vi "IE Default UI.vi"(10 "Color icon in":T4={"image type"=0, "image depth"=8, "image"=[255, 255, 255, 255, 255, 255, 255, 255, 255, 255, 255, 255, 255, 255, 255, 255, 255, 255, 255, 255, 255, 255, 255, 255, 255, 255, 255, 255, 255, 255, 255, 255, 255, 0, 0, 0, 0, 0, 0, 0, 0, 0, 0, 0, 0, 0, 0, 0, 0, 0, 0, 0, 0, 0, 0, 0, 0, 0, 0, 0, 0, 0, 0, 255, 255, 0, 0, 0, 0, 0, 0, 0, 0, 0, 0, 0, 0, 0, 0, 0, 0, 0, 0, 0, 0, 0, 0, 0, 0, 0, 0, 0, 0, 0, 0, 255, 255, 0, 0, 255, 255, 255, 255, 255, 255, 255, 255, 255, 255, 255, 255, 255, 255, 255, 255, 255, 255, 255, 0, 0, 0, 0, 0, 0, 0, 0, 0, 255, 255, 0, 0, 255, 250, 250, 250, 250, 250, 250, 250, 250, 250, 250, 250, 250, 248, 250, 44, 250, 44, 255, 0, 0, 0, 0, 0, 0, 0, 0, 0, 255, 255, 0, 0, 255, 250, 255, 255, 255, 255, 255, 255, 255, 255, 255, 255, 255, 248, 250, 44, 250, 44, 255, 0, 0, 0, 0, 0, 0, 0, 0, 0, 255, 255, 0, 0, 255, 250, 255, 209, 197, 209, 255, 255, 255, 209, 197, 209, 255, 248, 252, 43, 252, 44, 255, 0, 0, 0, 0, 0, 0, 0, 0, 0, 255, 255, 0, 0, 255, 250, 255, 197, 255, 197, 255, 255, 255, 197, 255, 197, 255, 248, 44, 44, 44, 44, 255, 0, 0, 0, 0, 0, 0, 0, 0, 0, 255, 255, 0, 0, 255, 250, 209, 197, 255, 197, 209, 255, 209, 197, 255, 197, 209, 248, 43, 252, 43, 44, 255, 0, 0, 0, 0, 0, 0, 0, 0, 0, 255, 255, 0, 0, 255, 250, 197, 209, 255, 209, 197, 255, 197, 209, 255, 209, 197, 248, 252, 8, 252, 44, 255, 0, 0, 0, 0, 0, 0, 0, 0, 0, 255, 255, 0, 0, 255, 250, 197, 255, 255, 255, 197, 255, 197, 255, 255, 255, 197, 248, 252, 8, 252, 44, 255, 0, 0, 0, 0, 0, 0, 0, 0, 0, 255, 255, 0, 0, 255, 250, 255, 255, 255, 255, 209, 197, 209, 255, 255, 255, 255, 248, 43, 252, 43, 44, 255, 0, 0, 0, 0, 0, 0, 0, 0, 0, 255, 255, 0, 0, 255, 250, 255, 255, 255, 255, 255, 255, 255, 255, 255, 255, 255, 248, 44, 44, 44, 44, 255, 0, 0, 0, 0, 0, 0, 0, 0, 0, 255, 255, 0, 0, 255, 248, 248, 248, 248, 248, 248, 248, 248, 248, 248, 248, 248, 248, 44, 44, 131, 131, 255, 0, 0, 0, 0, 0, 0, 0, 0, 0, 255, 255, 0, 0, 255, 44, 44, 44, 44, 44, 44, 44, 44, 44, 44, 44, 44, 44, 44, 44, 131, 5, 131, 131, 0, 0, 0, 0, 0, 0, 0, 0, 255, 255, 0, 0, 255, 44, 252, 44, 44, 44, 44, 44, 252, 44, 44, 44, 44, 35, 35, 35, 131, 5, 5, 5, 131, 131, 0, 0, 0, 0, 0, 0, 255, 255, 0, 0, 255, 252, 213, 252, 44, 44, 44, 252, 35, 252, 44, 35, 35, 44, 44, 44, 131, 5, 5, 255, 5, 5, 131, 131, 0, 0, 0, 0, 255, 255, 0, 0, 255, 44, 212, 44, 44, 44, 44, 35, 44, 44, 35, 44, 44, 44, 44, 44, 131, 5, 255, 255, 255, 5, 5, 5, 131, 35, 35, 0, 255, 255, 0, 0, 255, 255, 213, 255, 255, 255, 35, 255, 255, 35, 255, 255, 255, 255, 255, 255, 131, 5, 5, 255, 5, 5, 131, 131, 0, 0, 0, 0, 255, 255, 0, 0, 0, 0, 212, 0, 0, 0, 35, 0, 0, 35, 0, 0, 213, 212, 212, 213, 131, 5, 5, 5, 131, 131, 0, 0, 0, 0, 0, 0, 255, 255, 0, 0, 0, 0, 0, 213, 0, 0, 0, 35, 35, 0, 0, 212, 0, 0, 0, 0, 131, 5, 131, 131, 0, 0, 0, 0, 0, 0, 0, 0, 255, 255, 0, 0, 0, 0, 0, 0, 212, 212, 0, 0, 0, 0, 213, 0, 0, 0, 0, 0, 131, 131, 0, 0, 0, 0, 0, 0, 0, 0, 0, 0, 255, 255, 0, 0, 0, 0, 0, 0, 0, 0, 213, 212, 213, 212, 0, 0, 0, 0, 0, 0, 0, 0, 0, 0, 0, 0, 255, 255, 0, 0, 0, 0, 255, 255, 0, 0, 0, 0, 0, 0, 0, 0, 0, 0, 0, 0, 0, 0, 0, 0, 0, 0, 0, 0, 0, 0, 0, 255, 0, 0, 255, 0, 0, 0, 255, 255, 0, 0, 0, 0, 0, 0, 0, 0, 0, 0, 0, 0, 0, 0, 0, 0, 0, 0, 0, 0, 0, 0, 0, 0, 0, 0, 255, 0, 0, 0, 255, 255, 0, 0, 0, 0, 0, 0, 0, 0, 0, 0, 0, 0, 0, 0, 0, 0, 0, 0, 0, 0, 0, 0, 0, 0, 255, 255, 0, 0, 0, 0, 255, 255, 0, 0, 0, 0, 0, 0, 0, 0, 0, 0, 0, 0, 0, 0, 0, 0, 0, 0, 0, 0, 0, 0, 0, 0, 0, 0, 255, 0, 0, 0, 255, 255, 0, 0, 0, 0, 0, 0, 0, 0, 0, 0, 0, 0, 0, 0, 0, 0, 0, 0, 0, 0, 0, 0, 0, 255, 0, 0, 255, 0, 0, 0, 255, 255, 0, 0, 0, 0, 0, 0, 0, 0, 0, 0, 0, 0, 0, 0, 0, 0, 0, 0, 0, 0, 0, 0, 0, 0, 255, 255, 0, 0, 0, 0, 255, 255, 0, 0, 0, 0, 0, 0, 0, 0, 0, 0, 0, 0, 0, 0, 0, 0, 0, 0, 0, 0, 0, 0, 0, 0, 0, 0, 0, 0, 0, 0, 255, 255, 0, 0, 0, 0, 0, 0, 0, 0, 0, 0, 0, 0, 0, 0, 0, 0, 0, 0, 0, 0, 0, 0, 0, 0, 0, 0, 0, 0, 0, 0, 255, 255, 255, 255, 255, 255, 255, 255, 255, 255, 255, 255, 255, 255, 255, 255, 255, 255, 255, 255, 255, 255, 255, 255, 255, 255, 255, 255, 255, 255, 255, 255, 255], "mask"=[], "colors"=[16777215, 16777164, 16777113, 16777062, 16777011, 16776960, 16764159, 16764108, 16764057, 16764006, 16763955, 16763904, 16751103, 16751052, 16751001, 16750950, 16750899, 16750848, 16738047, 16737996, 16737945, 16737894, 16737843, 16737792, 16724991, 16724940, 16724889, 16724838, 16724787, 16724736, 16711935, 16711884, 16711833, 16711782, 16711731, 16711680, 13434879, 13434828, 13434777, 13434726, 13434675, 13434624, 13421823, 13421772, 13421721, 13421670, 13421619, 13421568, 13408767, 13408716, 13408665, 13408614, 13408563, 13408512, 13395711, 13395660, 13395609, 13395558, 13395507, 13395456, 13382655, 13382604, 13382553, 13382502, 13382451, 13382400, 13369599, 13369548, 13369497, 13369446, 13369395, 13369344, 10092543, 10092492, 10092441, 10092390, 10092339, 10092288, 10079487, 10079436, 10079385, 10079334, 10079283, 10079232, 10066431, 10066380, 10066329, 10066278, 10066227, 10066176, 10053375, 10053324, 10053273, 10053222, 10053171, 10053120, 10040319, 10040268, 10040217, 10040166, 10040115, 10040064, 10027263, 10027212, 10027161, 10027110, 10027059, 10027008, 6750207, 6750156, 6750105, 6750054, 6750003, 6749952, 6737151, 6737100, 6737049, 6736998, 6736947, 6736896, 6724095, 6724044, 6723993, 6723942, 6723891, 6723840, 6711039, 6710988, 6710937, 6710886, 6710835, 6710784, 6697983, 6697932, 6697881, 6697830, 6697779, 6697728, 6684927, 6684876, 6684825, 6684774, 6684723, 6684672, 3407871, 3407820, 3407769, 3407718, 3407667, 3407616, 3394815, 3394764, 3394713, 3394662, 3394611, 3394560, 3381759, 3381708, 3381657, 3381606, 3381555, 3381504, 3368703, 3368652, 3368601, 3368550, 3368499, 3368448, 3355647, 3355596, 3355545, 3355494, 3355443, 3355392, 3342591, 3342540, 3342489, 3342438, 3342387, 3342336, 65535, 65484, 65433, 65382, 65331, 65280, 52479, 52428, 52377, 52326, 52275, 52224, 39423, 39372, 39321, 39270, 39219, 39168, 26367, 26316, 26265, 26214, 26163, 26112, 13311, 13260, 13209, 13158, 13107, 13056, 255, 204, 153, 102, 51, 15597568, 14483456, 12255232, 11141120, 8912896, 7798784, 5570560, 4456448, 2228224, 1114112, 60928, 56576, 47872, 43520, 34816, 30464, 21760, 17408, 8704, 4352, 238, 221, 187, 170, 136, 119, 85, 68, 34, 17, 15658734, 14540253, 12303291, 11184810, 8947848, 7829367, 5592405, 4473924, 2236962, 1118481, 0], "Rectangle"={"left"=0, "top"=0, "right"=32, "bottom"=32}}, 11 "BW icon in":T4={"image type"=0, "image depth"=1, "image"=[255, 255, 255, 255, 128, 0, 0, 1, 128, 0, 0, 1, 159, 255, 252, 1, 144, 0, 84, 1, 151, 255, 84, 1, 150, 251, 84, 1, 149, 117, 4, 1, 149, 117, 36, 1, 147, 174, 84, 1, 147, 174, 84, 1, 151, 223, 36, 1, 151, 255, 4, 1, 144, 0, 28, 1, 144, 0, 22, 1, 148, 16, 241, 129, 158, 59, 18, 97, 148, 36, 23, 29, 159, 255, 242, 97, 132, 73, 241, 129, 130, 50, 22, 1, 129, 132, 24, 1, 128, 120, 0, 97, 128, 0, 0, 145, 128, 0, 0, 17, 128, 0, 0, 97, 128, 0, 0, 17, 128, 0, 0, 145, 128, 0, 0, 97, 128, 0, 0, 1, 128, 0, 0, 1, 255, 255, 255, 255], "mask"=[], "colors"=[16777215, 0], "Rectangle"={"left"=0, "top"=0, "right"=32, "bottom"=32}}) -> (0 "Error code out":i32=43, 2 "Color icon out":T4={"image type"=0, "image depth"=24, "image"=array[3072 elements], "mask"=[0, 0, 0, 0, 0, 0, 0, 0, 0, 0, 0, 0, 0, 0, 0, 0, 0, 0, 0, 0, 0, 0, 0, 0, 0, 0, 0, 0, 0, 0, 0, 0, 0, 0, 0, 0, 0, 0, 0, 0, 0, 0, 0, 0, 0, 0, 0, 0, 0, 0, 0, 0, 0, 0, 0, 0, 0, 0, 0, 0, 0, 0, 0, 0, 0, 0, 0, 0, 0, 0, 0, 0, 0, 0, 0, 0, 0, 0, 0, 0, 0, 0, 0, 0, 0, 0, 0, 0, 0, 0, 0, 0, 0, 0, 0, 0, 0, 0, 0, 0, 0, 0, 0, 0, 0, 0, 0, 0, 0, 0, 0, 0, 0, 0, 0, 0, 0, 0, 0, 0, 0, 0, 0, 0, 0, 0, 0, 0], "colors"=[], "Rectangle"={"left"=0, "top"=0, "right"=32, "bottom"=32}}, 3 "BW icon out":T4={"image type"=0, "image depth"=1, "image"=[0, 0, 0, 0, 0, 0, 0, 0, 0, 0, 0, 0, 0, 0, 0, 0, 0, 0, 0, 0, 0, 0, 0, 0, 0, 0, 0, 0, 0, 0, 0, 0, 0, 0, 0, 0, 0, 0, 0, 0, 0, 0, 0, 0, 0, 0, 0, 0, 0, 0, 0, 0, 0, 0, 0, 0, 0, 0, 0, 0, 0, 0, 0, 0, 0, 0, 0, 0, 0, 0, 0, 0, 0, 0, 0, 0, 0, 0, 0, 0, 0, 0, 0, 0, 0, 0, 0, 0, 0, 0, 0, 0, 0, 0, 0, 0, 0, 0, 0, 0, 0, 0, 0, 0, 0, 0, 0, 0, 0, 0, 0, 0, 0, 0, 0, 0, 0, 0, 0, 0, 0, 0, 0, 0, 0, 0, 0, 0], "mask"=[], "colors"=[16777215, 0], "Rectangle"={"left"=0, "top"=0, "right"=32, "bottom"=32}})   [LabVIEW 2021]
doc: "<p>Display this dialog box in one of the following ways:</p>\n\n<ul>\n<li>Double-click the <a href=\"nihelplauncher://docs/csh?context=lvcore_lvconcepts_using_icons\">icon</a> in the upper right corner of the front panel window, block diagram window, or <a href=\"nihelplauncher://docs/csh?context=lvcore_lvconcepts_custom_cont_ind_type\">Control Editor</a> window.</li>\n<li>Right-click the icon in the upper right corner of the front panel window, block diagram window, or <strong>Control Editor</strong> window and select <strong>Edit Icon</strong> from the shortcut menu.</li>\n<li>Select <strong>File<span class=\"U+187\">>></span>VI Properties</strong> or <strong>File<span class=\"U+187\">>></span>Control Properties</strong> to display the <a href=\"nihelplauncher://docs/csh?context=lvcore_lvdialog_vi_properties_dialog_box\">VI Properties</a> dialog box or <strong>Control Properties</strong> dialog box, respectively. Then select <strong>General</strong> from the <strong>Category</strong> pull-down menu and click the <strong>Edit Icon</strong> button.</li>\n<li>Right-click a project library, statechart, class, or XControl item in the <a href=\"nihelplauncher://docs/csh?context=lvcore_lvconcepts_using_labview_projects\">Project Explorer</a> window and select <strong> Properties</strong> from the shortcut menu to display the corresponding <strong>Properties</strong> dialog box. Then click the <strong>Edit</strong> button on the <strong>General Settings</strong> page.</li>\n</ul>\n\n<p>Use this dialog box to <a href=\"nihelplauncher://docs/csh?context=lvcore_lvhowto_creating_icons\">create and edit icons</a>.</p>"
uses:
  <vilib>/LabVIEW Icon API/lv_icon/Controls/BodyText.ctl
  <vilib>/LabVIEW Icon API/lv_icon/Controls/Font.ctl
  <vilib>/LabVIEW Icon API/lv_icon/Controls/Alignment.ctl
  <vilib>/LabVIEW Icon API/lv_icon/Controls/Layer.ctl
  <resource>/plugins/NIIconEditor/Controls/LayerList.ctl
  <resource>/plugins/NIIconEditor/Controls/NewLayer.ctl
  <resource>/plugins/NIIconEditor/Controls/DeleteLayer.ctl
  <resource>/plugins/NIIconEditor/Controls/Arrow Up.ctl
  <resource>/plugins/NIIconEditor/Controls/Arrow Down.ctl
  <resource>/plugins/NIIconEditor/Controls/Framework Templates.ctl
  <vilib>/LabVIEW Icon API/lv_icon/Controls/Graphic.ctl
  <resource>/plugins/NIIconEditor/Controls/ColorChange.ctl
  <vilib>/LabVIEW Icon API/lv_icon/Controls/IEColor.ctl
  <resource>/plugins/NIIconEditor/Controls/Rotate.ctl
  <resource>/plugins/NIIconEditor/Controls/Flip.ctl
  <resource>/plugins/NIIconEditor/Controls/Tools.ctl
  <resource>/plugins/NIIconEditor/Controls/Pen.ctl
  <resource>/plugins/NIIconEditor/Controls/Line.ctl
  <resource>/plugins/NIIconEditor/Controls/Dropper.ctl
  <resource>/plugins/NIIconEditor/Controls/Fill.ctl
  <resource>/plugins/NIIconEditor/Controls/IERect.ctl
  <resource>/plugins/NIIconEditor/Controls/FRect.ctl
  <resource>/plugins/NIIconEditor/Controls/Circle.ctl
  <resource>/plugins/NIIconEditor/Controls/FCircle.ctl
  <resource>/plugins/NIIconEditor/Controls/Rubber.ctl
  <resource>/plugins/NIIconEditor/Controls/Text.ctl
  <resource>/plugins/NIIconEditor/Controls/Selection.ctl
  <resource>/plugins/NIIconEditor/Controls/Move.ctl
  <resource>/plugins/NIIconEditor/Controls/TextMarker.ctl
  <vilib>/picture/picture.llb/imagedata.ctl
  <resource>/plugins/NIIconEditor/Controls/Path&Icon.ctl
  <resource>/plugins/NIIconEditor/Controls/Refresh.ctl
  <vilib>/Utility/miscctls.llb/LVKeyNavTypeDef.ctl
  <resource>/plugins/NIIconEditor/Controls/References Cluster.ctl
  <vilib>/Utility/miscctls.llb/LVPoint32TypeDef.ctl
  <vilib>/LabVIEW Icon API/lv_icon/Controls/Pathes.ctl
  <resource>/plugins/NIIconEditor/Class/Ants/Ants.lvclass
  <resource>/plugins/NIIconEditor/Class/FakedArray/FakedArray.lvclass
  <vilib>/LabVIEW Icon API/lv_icon/Classes/Icon/Icon.lvclass
  <resource>/plugins/NIIconEditor/Class/Icon Library/Glyph.lvclass
  <vilib>/LabVIEW Icon API/lv_icon/lv_icon.lvlib
  <resource>/dialog/lvconfig.llb/LV Config Read String.vi
  <resource>/dialog/lvconfig.llb/LV Config Write String.vi
panel:
  out "LabVIEW Icon out":string
  in  "LabVIEW Icon in":string
  out "Terminals":picture
  out "Preview2":picture
  in  "?":cluster{T1[], i32, bool}
  out "TextMarker":T2="^"
  in  "Help":bool
  in  "Cancel":bool
  in  "OK":bool
  out "XYZ":string="X: 14\nY: 31\nZ: 1"
  out "RGB":string="R: 0\nG: 0\nB: 0"
  out "Icon":picture
  out "Clipboard":picture
  in  "?":T3[](array[typedef])
  in  "Tab Control":T5(tab)
  in  "refreshTemplates":T6
  out "templates path str":string
  in  "Templates":string(tree)="<All>"
  in  "Filter templates by keyword":string
  in  "Framework Templates":T7={"Scrollbar"=0, "Path & Icon 1"={"Rectangle"={"left"=0, "top"=0, "right"=32, "bottom"=32}, "Path"=path "C:/Users/tsandris/Documents/LabVIEW Data/Icon Templates/VI/Frameworks/_blank.png", "Image"=bytes[3230], "Filter"="VI\\Frameworks", "FileName"="_blank"}, "Path & Icon 2"={"Rectangle"={"left"=0, "top"=0, "right"=32, "bottom"=32}, "Path"=path "C:/Users/tsandris/Documents/LabVIEW Data/Icon Templates/Library/Frameworks/_blank.png", "Image"=bytes[3230], "Filter"="Library\\Frameworks", "FileName"="_blank"}, "Path & Icon 3"={"Rectangle"={"left"=0, "top"=0, "right"=0, "bottom"=0}, "Path"=path "", "Image"=bytes[0], "Filter"="", "FileName"=""}, "Path & Icon 4"={"Rectangle"={"left"=0, "top"=0, "right"=0, "bottom"=0}, "Path"=path "", "Image"=bytes[0], "Filter"="", "FileName"=""}, "Path & Icon 5"={"Rectangle"={"left"=0, "top"=0, "right"=0, "bottom"=0}, "Path"=path "", "Image"=bytes[0], "Filter"="", "FileName"=""}, "Path & Icon 6"={"Rectangle"={"left"=0, "top"=0, "right"=0, "bottom"=0}, "Path"=path "", "Image"=bytes[0], "Filter"="", "FileName"=""}, "Path & Icon 7"={"Rectangle"={"left"=0, "top"=0, "right"=0, "bottom"=0}, "Path"=path "", "Image"=bytes[0], "Filter"="", "FileName"=""}, "Path & Icon 8"={"Rectangle"={"left"=0, "top"=0, "right"=0, "bottom"=0}, "Path"=path "", "Image"=bytes[0], "Filter"="", "FileName"=""}, "Path & Icon 9"={"Rectangle"={"left"=0, "top"=0, "right"=0, "bottom"=0}, "Path"=path "", "Image"=bytes[0], "Filter"="", "FileName"=""}, "Path & Icon 10"={"Rectangle"={"left"=0, "top"=0, "right"=0, "bottom"=0}, "Path"=path "", "Image"=bytes[0], "Filter"="", "FileName"=""}, "Path & Icon 11"={"Rectangle"={"left"=0, "top"=0, "right"=0, "bottom"=0}, "Path"=path "", "Image"=bytes[0], "Filter"="", "FileName"=""}, "Path & Icon 12"={"Rectangle"={"left"=0, "top"=0, "right"=0, "bottom"=0}, "Path"=path "", "Image"=bytes[0], "Filter"="", "FileName"=""}, "Path & Icon 13"={"Rectangle"={"left"=0, "top"=0, "right"=0, "bottom"=0}, "Path"=path "", "Image"=bytes[0], "Filter"="", "FileName"=""}, "Path & Icon 14"={"Rectangle"={"left"=0, "top"=0, "right"=0, "bottom"=0}, "Path"=path "", "Image"=bytes[0], "Filter"="", "FileName"=""}, "Path & Icon 15"={"Rectangle"={"left"=0, "top"=0, "right"=0, "bottom"=0}, "Path"=path "", "Image"=bytes[0], "Filter"="", "FileName"=""}, "Path & Icon 16"={"Rectangle"={"left"=0, "top"=0, "right"=0, "bottom"=0}, "Path"=path "", "Image"=bytes[0], "Filter"="", "FileName"=""}, "Path & Icon 17"={"Rectangle"={"left"=0, "top"=0, "right"=0, "bottom"=0}, "Path"=path "", "Image"=bytes[0], "Filter"="", "FileName"=""}, "Path & Icon 18"={"Rectangle"={"left"=0, "top"=0, "right"=0, "bottom"=0}, "Path"=path "", "Image"=bytes[0], "Filter"="", "FileName"=""}, "Path & Icon 19"={"Rectangle"={"left"=0, "top"=0, "right"=0, "bottom"=0}, "Path"=path "", "Image"=bytes[0], "Filter"="", "FileName"=""}, "Path & Icon 20"={"Rectangle"={"left"=0, "top"=0, "right"=0, "bottom"=0}, "Path"=path "", "Image"=bytes[0], "Filter"="", "FileName"=""}, "Path & Icon 21"={"Rectangle"={"left"=0, "top"=0, "right"=0, "bottom"=0}, "Path"=path "", "Image"=bytes[0], "Filter"="", "FileName"=""}, "Path & Icon 22"={"Rectangle"={"left"=0, "top"=0, "right"=0, "bottom"=0}, "Path"=path "", "Image"=bytes[0], "Filter"="", "FileName"=""}, "Path & Icon 23"={"Rectangle"={"left"=0, "top"=0, "right"=0, "bottom"=0}, "Path"=path "", "Image"=bytes[0], "Filter"="", "FileName"=""}, "Path & Icon 24"={"Rectangle"={"left"=0, "top"=0, "right"=0, "bottom"=0}, "Path"=path "", "Image"=bytes[0], "Filter"="", "FileName"=""}, "Path & Icon 25"={"Rectangle"={"left"=0, "top"=0, "right"=0, "bottom"=0}, "Path"=path "", "Image"=bytes[0], "Filter"="", "FileName"=""}, "Path & Icon 26"={"Rectangle"={"left"=0, "top"=0, "right"=0, "bottom"=0}, "Path"=path "", "Image"=bytes[0], "Filter"="", "FileName"=""}, "Path & Icon 27"={"Rectangle"={"left"=0, "top"=0, "right"=0, "bottom"=0}, "Path"=path "", "Image"=bytes[0], "Filter"="", "FileName"=""}, "Path & Icon 28"={"Rectangle"={"left"=0, "top"=0, "right"=0, "bottom"=0}, "Path"=path "", "Image"=bytes[0], "Filter"="", "FileName"=""}, "Path & Icon 29"={"Rectangle"={"left"=0, "top"=0, "right"=0, "bottom"=0}, "Path"=path "", "Image"=bytes[0], "Filter"="", "FileName"=""}, "Path & Icon 30"={"Rectangle"={"left"=0, "top"=0, "right"=0, "bottom"=0}, "Path"=path "", "Image"=bytes[0], "Filter"="", "FileName"=""}}
  in  "Body Text":T8={"Line 1 text"="", "Line 2 text"="", "Line 3 text"="", "Line 4 text"="", "Line 1 color"=0, "Line 2 color"=0, "Line 3 color"=0, "Line 4 color"=0, "Body Text Spec"={"Font"="", "Alignment"=1, "Size"=9}, "Center text vertically"=TRUE, "Capitalize Text"=TRUE} {"Body Text Spec"."Alignment" items=["left", "center", "right"]}
  in  "Filter glyphs by keyword":string
  in  "Glyphs":string(tree)="<All>"
  out "glyph path str":string
  out "Glyphs []":T1[][](array[typedef])
  in  "refreshGlyphs":T6
  in  "Add Layer":T11
  in  "Remove Layer":T12
  in  "Move Down":T13
  in  "Move Up":T14
  in  "Icon Template":T15={"LayerIcon"=bytes[0], "LayerName"="", "Opacity"=100, "Visibility?"=TRUE} {"Opacity" scale=0.0..100.0}
  in  "Icon Text":T15={"LayerIcon"=bytes[0], "LayerName"="Icon Text", "Opacity"=100, "Visibility?"=TRUE} {"Opacity" scale=0.0..100.0}
  in  "User Layers":T16={"Scrollbar"=0, "Layer 1"={"LayerIcon"=bytes[3230], "LayerName"="VI Icon", "Opacity"=100, "Visibility?"=TRUE}, "Layer 2"={"LayerIcon"=bytes[3230], "LayerName"="", "Opacity"=100, "Visibility?"=TRUE}, "Layer 3"={"LayerIcon"=bytes[3230], "LayerName"="", "Opacity"=100, "Visibility?"=TRUE}, "Layer 4"={"LayerIcon"=bytes[3230], "LayerName"="", "Opacity"=100, "Visibility?"=TRUE}} {"Layer 4"."Opacity" scale=0.0..100.0; "Layer 3"."Opacity" scale=0.0..100.0; "Layer 2"."Opacity" scale=0.0..100.0; "Layer 1"."Opacity" scale=0.0..100.0}
  out "Preview":picture
  in  "Horizontal Flip":T17
  in  "Clockwise Rotate":T18
  in  "Swap":T19
  in  "Line Color":T20
  in  "Fill Color":T20=16777215
  in  "Tools":T21=enum."Rectangle"
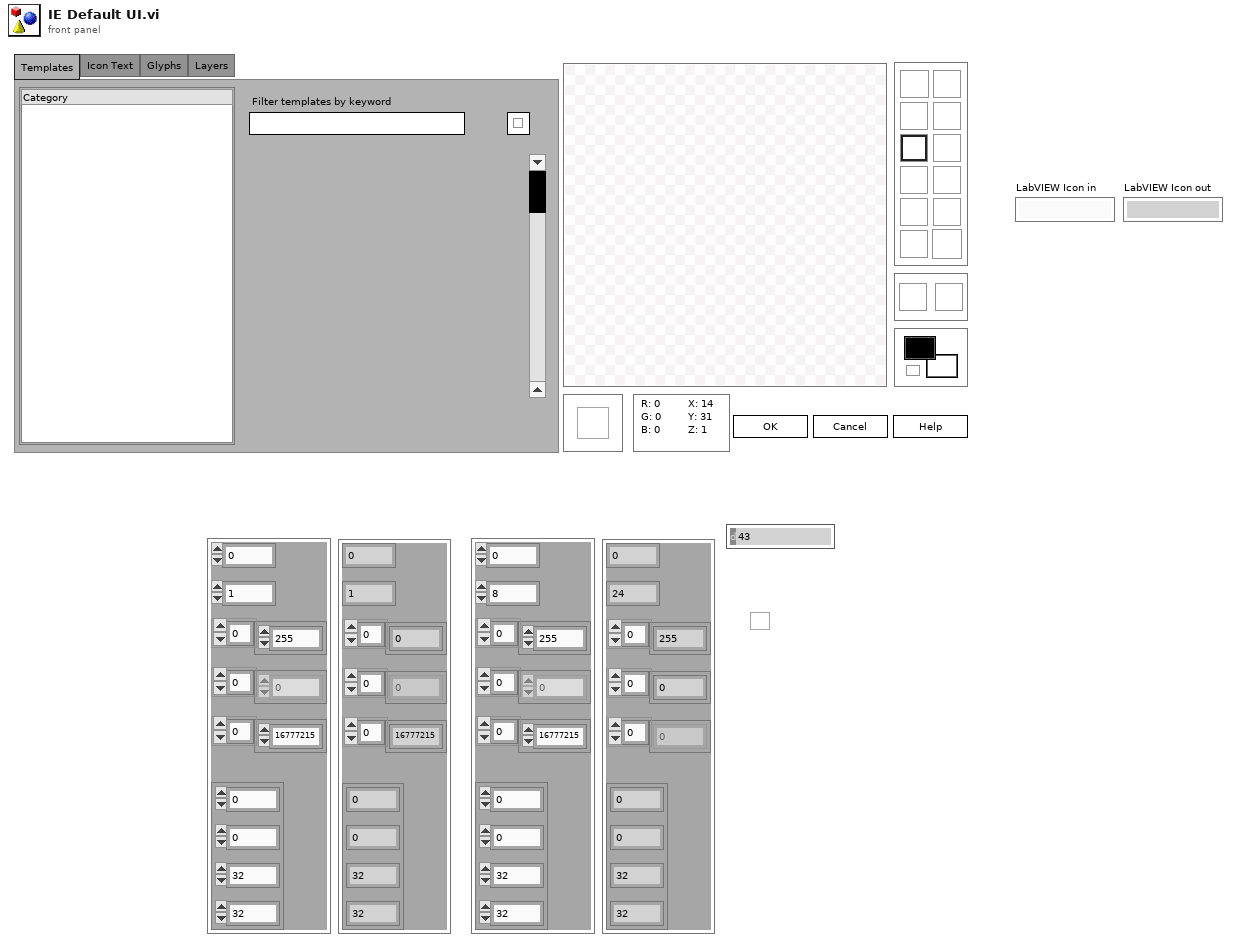
[diagram p1: front panel]
types:
  T1 = typedef "Graphic.ctl" = cluster{"Rectangle":cluster{"left":i16, "top":i16, "right":i16, "bottom":i16}, "Path":path, "Image":picture, "Filter":string, "FileName":string}
  T2 = typedef "TextMarker.ctl" = string
  T3 = typedef "Path&Icon.ctl" = cluster{"Rectangle":cluster{"left":i16, "top":i16, "right":i16, "bottom":i16}, "Path":path, "Image":picture, "Filter":string, "FileName":string}
  T4 = typedef "imagedata.ctl" = cluster{"image type":i32, "image depth":i32, "image":u8[], "mask":u8[], "colors":u32[], "Rectangle":cluster{"left":i16, "top":i16, "right":i16, "bottom":i16}}
  T5 = enum32{"Templates", "Icon Text", "Glyphs", "Layers"}
  T6 = typedef "Refresh.ctl" = bool
  T7 = typedef "Framework Templates.ctl" = cluster{"Scrollbar":i32, "Path & Icon 1":T1, "Path & Icon 2":T1, "Path & Icon 3":T1, "Path & Icon 4":T1, "Path & Icon 5":T1, "Path & Icon 6":T1, "Path & Icon 7":T1, "Path & Icon 8":T1, "Path & Icon 9":T1, "Path & Icon 10":T1, "Path & Icon 11":T1, "Path & Icon 12":T1, "Path & Icon 13":T1, "Path & Icon 14":T1, "Path & Icon 15":T1, "Path & Icon 16":T1, "Path & Icon 17":T1, "Path & Icon 18":T1, "Path & Icon 19":T1, "Path & Icon 20":T1, "Path & Icon 21":T1, "Path & Icon 22":T1, "Path & Icon 23":T1, "Path & Icon 24":T1, "Path & Icon 25":T1, "Path & Icon 26":T1, "Path & Icon 27":T1, "Path & Icon 28":T1, "Path & Icon 29":T1, "Path & Icon 30":T1}
  T8 = typedef "BodyText.ctl" = cluster{"Line 1 text":string, "Line 2 text":string, "Line 3 text":string, "Line 4 text":string, "Line 1 color":u32, "Line 2 color":u32, "Line 3 color":u32, "Line 4 color":u32, "Body Text Spec":cluster{"Font":T9, "Alignment":T10, "Size":u8}, "Center text vertically":bool, "Capitalize Text":bool}
  T9 = typedef "Font.ctl" = string
  T10 = typedef "Alignment.ctl" = u16
  T11 = typedef "NewLayer.ctl" = bool
  T12 = typedef "DeleteLayer.ctl" = bool
  T13 = typedef "Arrow Down.ctl" = bool
  T14 = typedef "Arrow Up.ctl" = bool
  T15 = typedef "Layer.ctl" = cluster{"LayerIcon":picture, "LayerName":string, "Opacity":u8, "Visibility?":bool}
  T16 = typedef "LayerList.ctl" = cluster{"Scrollbar":i32, "Layer 1":T15, "Layer 2":T15, "Layer 3":T15, "Layer 4":T15}
  T17 = typedef "Flip.ctl" = bool
  T18 = typedef "Rotate.ctl" = bool
  T19 = typedef "ColorChange.ctl" = bool
  T20 = typedef "IEColor.ctl" = u32
  T21 = typedef "Tools.ctl" = enum32{"Pencil", "Line", "Dropper", "Fill", "Rectangle", "Filled Rectangle", "Ellipse", "Filled Ellipse", "Eraser", "Text", "Select", "Move"}
  T22 = enum32{"Invalid", "Standard", "Closed", "Hidden", "Minimized", "Maximized"}
  T23 = typedef "References Cluster.ctl" = cluster{"Add Layer":refnum<vi>, "Remove Layer":refnum<vi>, "Line Text":refnum<vi>[], "Body Text Spec":refnum<vi>, "DNL_Font":refnum<vi>, "glyph path str":refnum<vi>, "templates path str":refnum<vi>, "Arrow Up":refnum<vi>, "Arrow Down":refnum<vi>, "IE VI Ref":refnum<vi>, "Glyphs tree":refnum<vi>, "Templates tree":refnum<vi>, "Layer Icon Text":refnum<vi>, "Layer Template":refnum<vi>, "Clipboard":refnum<vi>, "BW icon in":refnum<vi>, "Color icon in":refnum<vi>, "Layer Clust":refnum<vi>, "Body Text":refnum<vi>, "DNL_Framework Templates":refnum<vi>, "Search Templates":refnum<vi>, "TextMarker":refnum<vi>, "Tab Control":refnum<vi>, "Search Glyphs":refnum<vi>, "Line Color":refnum<vi>, "DNL_Glyphs []":refnum<vi>, "Fill Color":refnum<vi>, "Tools":refnum<vi>, "Glyphs tree":refnum<vi>, "Icon":refnum<vi>, "Preview":refnum<vi>, "Ants":refnum<vi>, "Terminals":refnum<vi>, "menu reference":refnum<k9>, "LayerNames":refnum<vi>[], "GlyphLoadAnimation":refnum<vi>, "TemplateLoadAnimation":refnum<vi>, "refreshGlyphs":refnum<vi>, "refreshTemplates":refnum<vi>}
  T24 = typedef "LVKeyNavTypeDef.ctl" = cluster{"Control":bool, "Shift":bool, "Key":string}
  T25 = cluster{"Left":i16, "Top":i16, "Right":i16, "Bottom":i16}
  T26 = typedef "LVAllMonitorsDisplayTypeDef.ctl" = cluster{"Bounds":cluster{"Left":i16, "Top":i16, "Right":i16, "Bottom":i16}, "Depth":i16}[]
  T27 = cluster{"Global stop?":refnum<user-event>, "Templates":refnum<user-event>, "Glyphs":refnum<user-event>}
  T28 = typedef "IE Data.ctl" = cluster{"Class":T29, "Ref":T23, "Support":T30}
  T29 = typedef "IE Classes.ctl" = cluster{"Ants":refnum<class "Ants.lvclass">, "Layer":refnum<class "FakedArray.lvclass">, "Templates":refnum<class "FakedArray.lvclass">, "Icon":refnum<class "Icon.lvclass">, "Glyph":refnum<class "Glyph.lvclass">, "Settings":refnum<class "Settings.lvclass">, "Tools":refnum<class "Tools Paint.lvclass">}
  T30 = typedef "SupportClass.ctl" = cluster{"AntsRect":cluster{"left":i16, "top":i16, "right":i16, "bottom":i16}, "Mouse Move Coords":T31, "Mouse Down Coords":T31, "Temp Coord":T31, "Action":T32, "Edge Color":T20, "Fill Color":T20, "Mouse Down?":bool, "Draft Mode?":bool, "Temp Icon":picture, "CTRL Pressed":bool, "Move Selection?":bool, "AntsRect Orig":cluster{"left":i16, "top":i16, "right":i16, "bottom":i16}, "Text":string, "TM Set?":bool, "Mouse inside icon?":bool, "Tool (old value)":u32, "Pencil Move Color":u32, "Swap Colors?":bool, "Shift pressed?":bool}
  T31 = typedef "LVPoint32TypeDef.ctl" = cluster{"Horizontal":i32, "Vertical":i32}
  T32 = typedef "SupportClass_Action.ctl" = enum16{"Default", "Move Selection", "Glyph Library", "Tool"}
  T33 = typedef "Pathes.ctl" = enum16{"Root Path", "Icon Templates", "Icon Templates VI", "Icon Templates Lib", "Glyphs"}
  T34 = typedef "lveventtype.ctl" = enum32{"Null", "Timeout", "Annotation Menu Selection", "Annotation Menu Selection?", "App Instance Close", "App Instance Close?", "Autoscale Range Change", "Bookmark Info Change", "Cell Edit", "Cell Edit?", "Cursor Grab", "Cursor Grab?", "Cursor Menu Selection", "Cursor Menu Selection?", "Cursor Move", "Cursor Release", "Data Change", "Direction Change", "Display State Change", "Drag Ended", "Drag Enter", "Drag Leave", "Drag Over", "Drag Source Update", "Drag Starting", "Drag Starting?", "Drop", "Exec State Change", "Key Down", "Key Down?", "Key Repeat", "Key Repeat?", "Key Up", "Listbox Double Click", "Menu Activation?", "Menu Selection (App)", "Menu Selection? (App)", "Menu Selection (User)", "Mouse Down", "Mouse Down?", "Mouse Enter", "Mouse Leave", "Mouse Move", "Mouse Up", "Mouse Wheel", "NI Security User Change (App)", "Pane Size", "Panel Close", "Panel Close?", "Panel Resize", "Plot Attribute Change", "Scale Range Change", "Shortcut Menu Activation?", "Shortcut Menu Selection (App)", "Shortcut Menu Selection? (App)", "Shortcut Menu Selection (User)", "Tree Double Click", "Tree Drag", "Tree Drag?", "Tree Drop", "Tree Drop?", "Tree Item Close", "Tree Item Close?", "Tree Item Open", "Tree Item Open?", "User Event", "Value Change"}
  T35 = typedef "eventvkey.ctl" = enum16{"ASCII", "Enter", "Return", "Shift", "Ctrl", "Alt", "Cmd", "Opt", "Caps", "NumLock", "Clear", "Break", "Up", "Down", "Left", "Right", "Insert", "Delete", "Home", "End", "PageUp", "PageDown", "Escape", "Help", "Pause", "ScrollLock", "F1", "F2", "F3", "F4", "F5", "F6", "F7", "F8", "F9", "F10", "F11", "F12", "F13", "F14", "F15", "F16", "F17", "F18", "F19", "F20", "F21", "F22", "F23", "F24", "Play", "VolumeUp", "VolumeDown", "Mute", "Two Byte Char"}
  T36 = cluster{"Shift":bool, "Ctrl":bool, "Alt":bool, "Cmd":bool, "Opt":bool}
  T37 = typedef "LVRectTypeDef.ctl" = cluster{"Left":i16, "Top":i16, "Right":i16, "Bottom":i16}
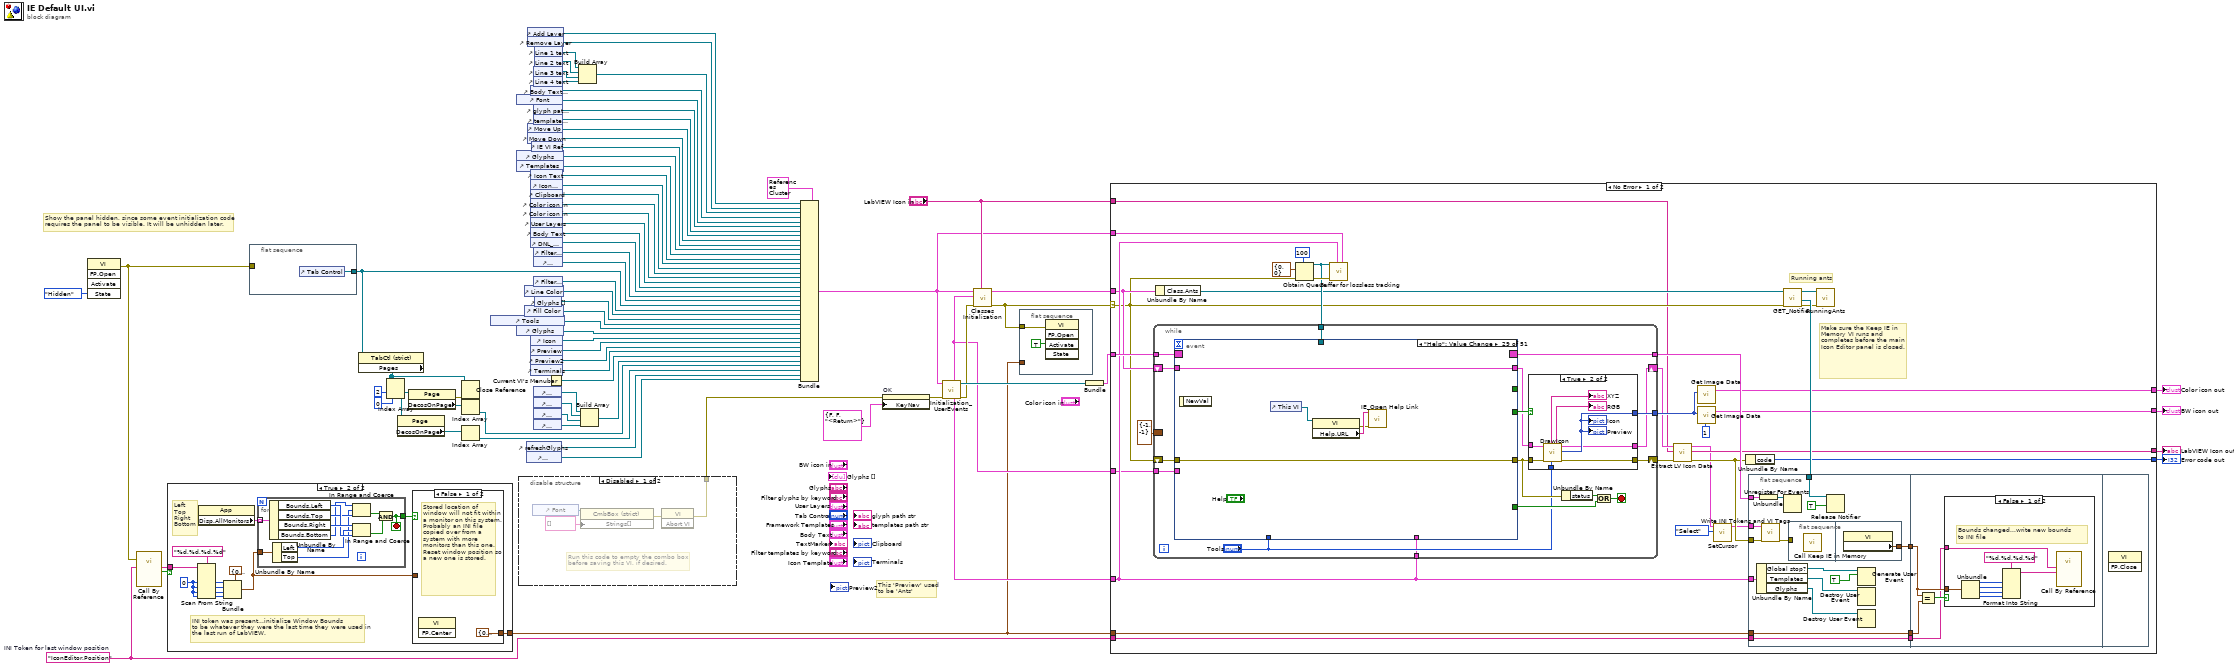
[diagram p0: block diagram]
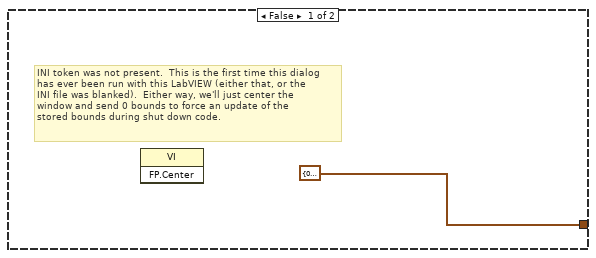
[diagram p2: hidden frame]
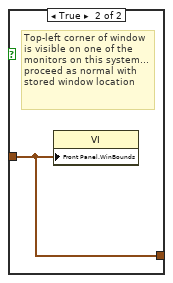
[diagram p3: hidden frame]
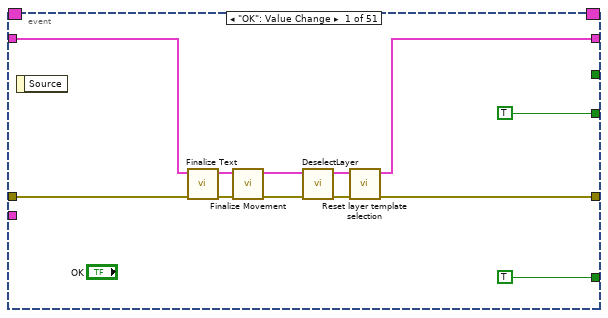
[diagram p6: hidden frame]
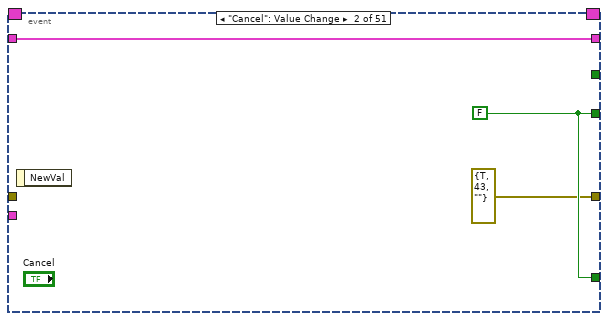
[diagram p7: hidden frame]
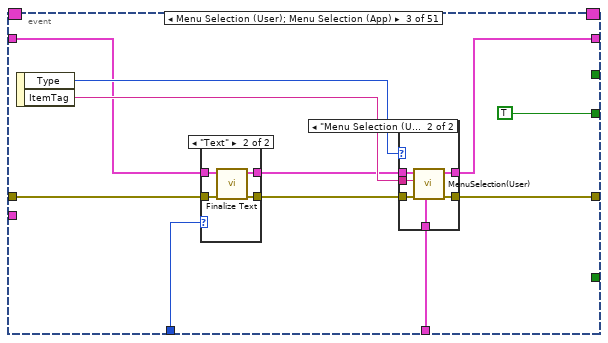
[diagram p8: hidden frame]
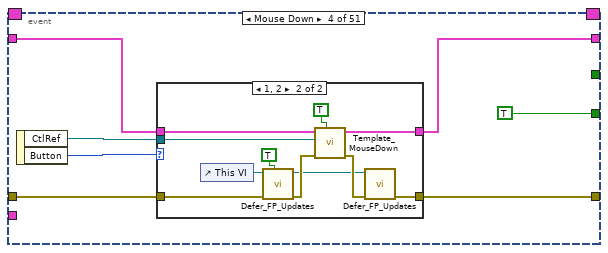
[diagram p11: hidden frame]
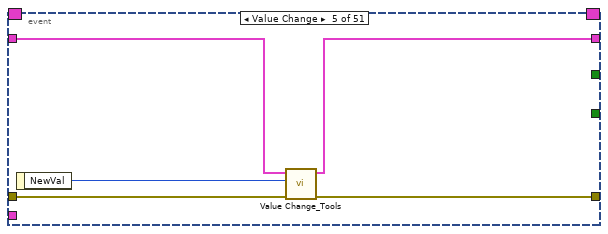
[diagram p13: hidden frame]
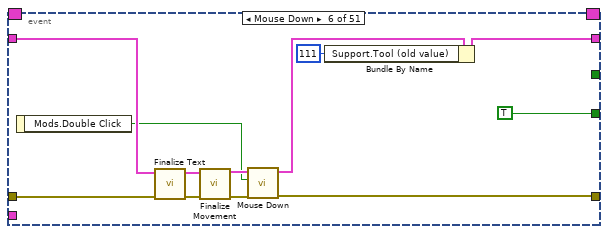
[diagram p14: hidden frame]
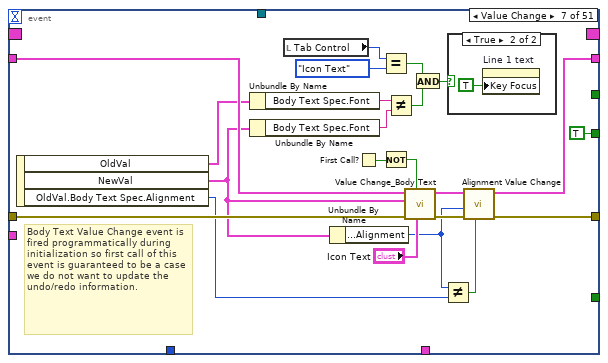
[diagram p15: hidden frame]
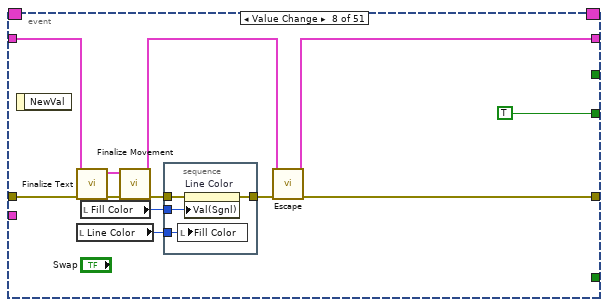
[diagram p17: hidden frame]
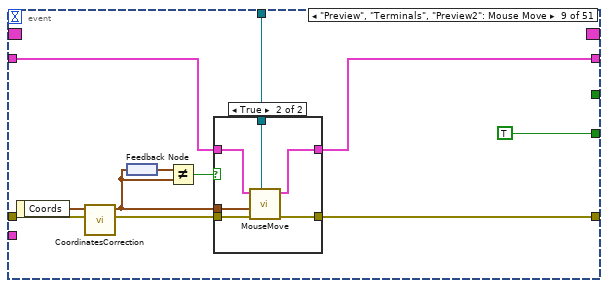
[diagram p18: hidden frame]
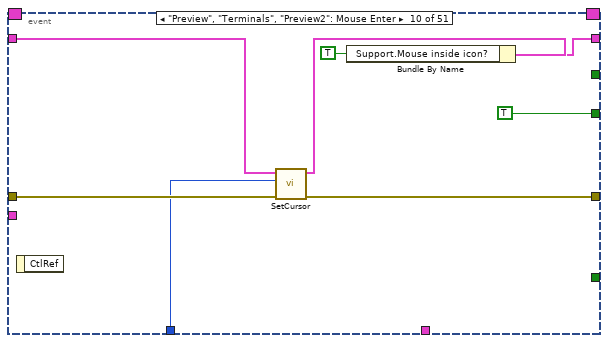
[diagram p20: hidden frame]
diagram:
  w1 = "IconEditor.Position"  # INI Token for last window position
  # "Show the panel hidden, since some event initialization code requires the panel to be visible. It will be unhidden later."
  # "This 'Preview' used\nto be 'Ants'"
  n1 = invoke class="VI" method="FP.Open"("State"=T22."Hidden") -> (error out=w3:errorcluster)  [unwired: 4 in, 4 out]
  n2 = call-by-ref "?"(error in=w3, "key"=w1) -> ("found?"=w4:bool, "value"=w5:string)  [unwired: 5 in, 3 out]
  n3 = case shown="True" w4 {
    tunnel: [T25 {"Left"=0, "Top"=0, "Right"=0, "Bottom"=0} ("Front Panel.PanelBounds") w79] -> w2
    tunnel: w5 -> [_ w90]
    frame False {
      # "INI token was not present.  This is the first time this dialog\nhas ever been run with this LabVIEW (either that, or the\nINI file was blanked).  Either way, we'll just center the\nwindow and send 0 bounds to force an update of the\nstored bounds during shut down code."
      n4 = invoke class="VI" method="FP.Center"() -> ()  [unwired: 3 in, 3 out]
    }
    frame True {
      w88 = i16 0 ("default value 1")
      # "Left\nTop\nRight\nBottom"
      # "INI token was present...initialize Window Bounds\nto be whatever they were the last time they were used in\nthe last run of LabVIEW."
      n5 = Scan From String(format string="%d,%d,%d,%d", input string=w90, default 1=w88, default 2=w88, default 3=w88, default 4=w88) -> (output 1=w87:i16, output 2=w86:i16, output 3=w85:i16, output 4=w84:i16)  [unwired: 2 in, 3 out]
      n6 = property class="App"() -> ("Disp.AllMonitors"=w82:T26)  [unwired: 2 in, 2 out]
      n7 = Bundle(cluster=T25 {"Left"=0, "Top"=0, "Right"=0, "Bottom"=0} ("Front Panel.PanelBounds"), "Left"=w87, "Top"=w86, "Right"=w85, "Bottom"=w84) -> (w81:T25)
      n8 = for {
        tunnel: w82 -> [w103] mode=indexing
        tunnel: w81 -> [w102]
        tunnel: [w93] -> w80
        stop <- w93 stop-if-true
        n9 = Unbundle By Name(w103) -> ("Bounds.Left"=w100:i16, "Bounds.Top"=w98:i16, "Bounds.Right"=w101:i16, "Bounds.Bottom"=w97:i16)
        n10 = Unbundle By Name(w102) -> ("Left"=w99:i16, "Top"=w96:i16)
        n11 = In Range and Coerce(upper limit=w97, x=w96, lower limit=w98) -> (In Range?=w95:bool)  [unwired: 1 out]
        n12 = In Range and Coerce(upper limit=w101, x=w99, lower limit=w100) -> (In Range?=w94:bool)  [unwired: 1 out]
        n13 = And(x=w95, y=w94) -> (x .and. y?=w93:bool)
      }
      n14 = case shown="False" w80 {
        tunnel: w81 -> [_ w92]
        tunnel: [T25 {"Left"=0, "Top"=0, "Right"=0, "Bottom"=0} ("Front Panel.PanelBounds") w92] -> w79
        frame False {
          # "Stored location of window will not fit within a monitor on this system.  Probably an INI file copied over from a system with more monitors than this one.  Reset window position so a new one is stored."
          n15 = invoke class="VI" method="FP.Center"() -> ()  [unwired: 3 in, 3 out]
        }
        frame True {
          # "Top-left corner of window is visible on one of the monitors on this system... proceed as normal with stored window location"
          n16 = property class="VI"("Front Panel.WinBounds"=w92) -> ()  [unwired: 2 in, 2 out]
        }
      }
    }
  }
  n17 = flat-sequence {
    tunnel: [w104] -> w18
    tunnel: w3 -> [_]
    frame #0 {
      n18 = control-ref of="Tab Control"() -> (w104:refnum<vi>)
    }
  }
  n19 = property class="TabCtl (strict)"(reference=w18) -> ("Pages"=w8:refnum<vi>[])  [unwired: 1 in, 2 out]
  n20 = Index Array(array=w8, index #1=2 ("index"), index #2=0 ("index")) -> (element #1=w14:refnum<vi>, element #2=w15:refnum<vi>)
  n21 = property class="Page"(reference=w15) -> ("DecosOnPage"=w12:refnum<vi>[])  [unwired: 1 in, 2 out]
  n22 = property class="Page"(reference=w14) -> (error out=w9:errorcluster, "DecosOnPage"=w13:refnum<vi>[])  [unwired: 1 in, 1 out]
  n23 = Close Reference(reference=w8, error in (no error)=w9) -> ()  [unwired: 1 out]
  n24 = Index Array(array=w13) -> (element=w10:refnum<vi>)  [unwired: 1 in]
  n25 = Index Array(array=w12) -> (element=w11:refnum<vi>)  [unwired: 1 in]
  n26 = control-ref of="Tools"() -> (w75:refnum<vi>)
  n27 = control-ref of="Glyphs"() -> (w53:refnum<vi>)
  n28 = control-ref of="Templates"() -> (w54:refnum<vi>)
  n29 = control-ref of="Glyphs"() -> (w55:refnum<vi>)
  n30 = control-ref of="Font"() -> (w32:refnum<vi>)
  n31 = disable-structure shown="Disabled" {
    disable-tunnel: [w105 _] -> w23
    frame Disabled {
      # "Run this code to empty the combo box\nbefore saving this VI, if desired."
      n32 = control-ref of="Font"() -> (w108:refnum<vi>)
      n33 = property class="CmbBox (strict)"(reference=w108, "Strings[]"=string[] [] ("Strings []")) -> (error out=w106:errorcluster)  [unwired: 1 in, 1 out]
      n34 = invoke class="VI" method="Abort VI"(error in=w106) -> (error out=w105:errorcluster)  [unwired: 2 in, 2 out]
    }
    frame Enabled {
    }
  }
  n35 = control-ref of="Line Color"() -> (w73:refnum<vi>)
  n36 = control-ref of="Fill Color"() -> (w74:refnum<vi>)
  n37 = control-ref of="refreshGlyphs"() -> (w19:refnum<vi>)
  n38 = control-ref of="refreshTemplates"() -> (w20:refnum<vi>)
  n39 = control-ref of="Move Up"() -> (w50:refnum<vi>)
  n40 = control-ref of="Move Down"() -> (w51:refnum<vi>)
  n41 = control-ref of="Add Layer"() -> (w38:refnum<vi>)
  n42 = control-ref of="Remove Layer"() -> (w39:refnum<vi>)
  n43 = control-ref of="Body Text Spec"() -> (w47:refnum<vi>)
  n44 = control-ref of="Icon Text"() -> (w57:refnum<vi>)
  n45 = control-ref of="Icon Template"() -> (w58:refnum<vi>)
  n46 = control-ref of="Color icon in"() -> (w35:refnum<vi>)
  n47 = control-ref of="Color icon in"() -> (w62:refnum<vi>)
  n48 = control-ref of="User Layers"() -> (w64:refnum<vi>)
  n49 = control-ref of="Body Text"() -> (w66:refnum<vi>)
  n50 = control-ref of="DNL_Framework Templates"() -> (w69:refnum<vi>)
  n51 = control-ref of="Clipboard"() -> (w60:refnum<vi>)
  n52 = control-ref of="Icon"() -> (w76:refnum<vi>)
  n53 = control-ref of="Preview"() -> (w77:refnum<vi>)
  n54 = control-ref of="Preview2"() -> (w46:refnum<vi>)
  n55 = control-ref of="Terminals"() -> (w65:refnum<vi>)
  n56 = control-ref of="IE VI Ref"() -> (w52:refnum<vi>)
  n57 = control-ref of="LayerName"() -> (w26:refnum<vi>)
  n58 = control-ref of="LayerName"() -> (w27:refnum<vi>)
  n59 = control-ref of="LayerName"() -> (w28:refnum<vi>)
  n60 = control-ref of="LayerName"() -> (w29:refnum<vi>)
  n61 = control-ref of="Line 3 text"() -> (w43:refnum<vi>)
  n62 = control-ref of="Line 4 text"() -> (w44:refnum<vi>)
  n63 = control-ref of="glyph path str"() -> (w48:refnum<vi>)
  n64 = control-ref of="templates path str"() -> (w49:refnum<vi>)
  n65 = control-ref of="Filter templates by keyword"() -> (w70:refnum<vi>)
  n66 = control-ref of="TextMarker"() -> (w71:refnum<vi>)
  n67 = control-ref of="Filter glyphs by keyword"() -> (w72:refnum<vi>)
  n68 = control-ref of="Line 1 text"() -> (w41:refnum<vi>)
  n69 = control-ref of="Line 2 text"() -> (w42:refnum<vi>)
  n70 = control-ref of="Glyphs []"() -> (w36:refnum<vi>)
  n71 = Current VI's Menubar() -> (w63:refnum<k9>)
  n72 = Build Array(w41, w42, w43, w44) -> (w40:refnum<vi>[])
  n73 = Build Array(w26, w27, w28, w29) -> (w24:refnum<vi>[])
  n74 = Bundle(cluster=T23 {"Add Layer"=refnum, "Remove Layer"=refnum, "Line Text"=[], "Body Text Spec"=refnum, "DNL_Font"=refnum, "glyph path str"=refnum, "templates path str"=refnum, "Arrow Up"=refnum, "Arrow Down"=refnum, "IE VI Ref"=refnum, "Glyphs tree"=refnum, "Templates tree"=refnum, "Layer Icon Text"=refnum, "Layer Template"=refnum, "Clipboard"=refnum, "BW icon in"=refnum, "Color icon in"=refnum, "Layer Clust"=refnum, "Body Text"=refnum, "DNL_Framework Templates"=refnum, "Search Templates"=refnum, "TextMarker"=refnum, "Tab Control"=refnum, "Search Glyphs"=refnum, "Line Color"=refnum, "DNL_Glyphs []"=refnum, "Fill Color"=refnum, "Tools"=refnum, "Glyphs tree"=refnum, "Icon"=refnum, "Preview"=refnum, "Ants"=refnum, "Terminals"=refnum, "menu reference"=refnum, "LayerNames"=[], "GlyphLoadAnimation"=refnum, "TemplateLoadAnimation"=refnum, "refreshGlyphs"=refnum, "refreshTemplates"=refnum} ("references"), "Add Layer"=w38, "Remove Layer"=w39, "Line Text"=w40, "Body Text Spec"=w47, "DNL_Font"=w32, "glyph path str"=w48, "templates path str"=w49, "Arrow Up"=w50, "Arrow Down"=w51, "IE VI Ref"=w52, "Glyphs tree"=w53, "Templates tree"=w54, "Layer Icon Text"=w57, "Layer Template"=w58, "Clipboard"=w60, "BW icon in"=w35, "Color icon in"=w62, "Layer Clust"=w64, "Body Text"=w66, "DNL_Framework Templates"=w69, "Search Templates"=w70, "TextMarker"=w71, "Tab Control"=w18, "Search Glyphs"=w72, "Line Color"=w73, "DNL_Glyphs []"=w36, "Fill Color"=w74, "Tools"=w75, "Glyphs tree"=w55, "Icon"=w76, "Preview"=w77, "Ants"=w46, "Terminals"=w65, "menu reference"=w63, "LayerNames"=w24, "GlyphLoadAnimation"=w10, "TemplateLoadAnimation"=w11, "refreshGlyphs"=w19, "refreshTemplates"=w20) -> (w25:T23)
  n75 = property on="OK" class="Bool"(error in=w23, "KeyNav"=T24 {"Control"=FALSE, "Shift"=FALSE, "Key"="<Return>"} ("Key Navigation")) -> (error out=w33:errorcluster)  [unwired: 1 in, 1 out]
  n76 = call <resource>:"Initialization_UserEvents.vi"("error in (no error)"=w33, "References"=w25) -> ("error out"=w59:errorcluster, "Events"=w68:refnum<event-registration>, "User events"=w22:T27)  [unwired: 7 out]
  n77 = call <resource>:"Classes Initialization.vi"("LabVIEW Icon in"="LabVIEW Icon in", "error in (no error)"=w59, "User events"=w22, "Ref Cluster"=w25) -> ("error out"=w7:errorcluster, "Data out"=w45:T28)  [unwired: 1 in, 5 out]
  n78 = flat-sequence {
    tunnel: w7 -> [w109]
    tunnel: w2 -> [_]
    frame #0 {
      n79 = invoke class="VI" method="FP.Open"(error in=w109, "Activate"=TRUE ("Activate?")) -> ()  [unwired: 3 in, 5 out]
    }
  }
  n80 = Bundle("Events"=w68) -> (w67:cluster{"Events":refnum<event-registration>})  [unwired: 1 in]
  n81 = case shown="No Error" w7 {
    selector: w7 -> [w125 w832]
    tunnel: w67 -> [w143 _]
    tunnel: [w141 w833] -> w61
    tunnel: [w138 _] -> w56
    tunnel: w22 -> [w131 _]
    tunnel: w45 -> [w130 _]
    tunnel: w25 -> [w128 _]
    tunnel: [w127 _] -> w37
    tunnel: "LabVIEW Icon in" -> [w120 w831]
    tunnel: [w123 w831] -> w30
    tunnel: w22 -> [w116 _]
    tunnel: w2 -> [w115 _]
    tunnel: w1 -> [w111 _]
    frame No Error {
      # "Make sure the Keep IE in Memory VI runs and completes before the main Icon Editor panel is closed."
      # "Running ants"
      n82 = Unbundle By Name(w130) -> ("Class.Ants"=w129:refnum<class "Ants.lvclass">)
      n83 = Obtain Queue(max queue size (-1, unlimited)=100, element data type=T31 {"Horizontal"=0, "Vertical"=0} ("Coords"), error in (no error)=w125) -> (queue out=w132:refnum<queue>, error out=w133:errorcluster)  [unwired: 1 in, 2 out]
      n84 = while {
        shift-right: [w153] -> w122
        shift-left: w125 -> [w161]
        tunnel: [w157] -> w144
        tunnel: w143 -> [w156]
        tunnel: [w155] -> w140
        tunnel: w132 -> [w150]
        tunnel: w131 -> [w149]
        shift-right: [w146] -> w124
        shift-left: w130 -> [w148]
        border: T31 {"Horizontal"=-1, "Vertical"=-1} ("Corrected Out") -> [_]
        tunnel: w116 -> [w145]
        stop <- w158 stop-if-true
        n85 = event shown="[28] \"Help\": Value Change" {
          selector: w156 -> [_ _ _ _ _ _ _ _ _ _ _ _ _ _ _ _ _ _ _ _ _ _ _ _ _ _ _ _ _ _ _ _ _ _ _ _ _ _ _ _ _ _ _ _ _ _ _ _ _ _ _]
          dyn-events: [_ _ _ _ _ _ _ _ _ _ _ _ _ _ _ _ _ _ _ _ _ _ _ _ _ _ _ _ _ _ _ _ _ _ _ _ _ _ _ _ _ _ _ _ _ _ _ _ _ _ _] -> w157
          timeout: _ -> [_ _ _ _ _ _ _ _ _ _ _ _ _ _ _ _ _ _ _ _ _ _ _ _ _ _ _ _ _ _ _ _ _ _ _ _ _ _ _ _ _ _ _ _ _ _ _ _ _ _ _]
          tunnel: [w177 errorcluster {"status"=TRUE, "code"=43, "source"=""} ("error out") w193 w216 w234 w238 w258 w280 w296 w312 w316 w330 w348 w355 w365 w373 w383 w393 w409 w417 w436 w450 w458 w476 w491 w506 w519 w537 w557 w564 w580 w590 w601 w604 w613 w627 w636 w648 w665 w675 w686 w689 w698 w711 errorcluster {"status"=TRUE, "code"=43, "source"=""} ("error out") w735 w765 w781 w786 w793 w800] -> w154
          tunnel: w161 -> [w179 _ w195 w218 w236 w243 w270 w274 w297 w313 w319 w331 w349 w354 w364 w375 w386 w401 w413 w426 w443 w451 w463 w481 w494 w512 w533 w545 w557 w563 w581 w593 w601 w605 w622 w630 w639 w650 w669 w676 w686 w690 w702 w714 _ w741 w769 w782 w787 w794 w801]
          tunnel: [TRUE w186 _ _ _ _ _ _ _ _ _ _ _ _ _ _ _ _ _ _ _ _ _ _ _ _ _ _ _ _ _ _ _ _ _ _ _ _ _ _ _ _ _ _ w729 _ _ _ _ _ _] -> w159
          tunnel: "Tools" -> [_ _ w189 _ _ _ _ _ _ w311 _ _ _ _ _ _ _ _ _ _ _ _ _ _ _ _ _ _ _ _ _ _ _ _ _ _ _ _ _ _ _ _ _ _ _ _ _ _ _ _ _]
          tunnel: [TRUE w186 TRUE TRUE _ TRUE TRUE TRUE TRUE TRUE TRUE TRUE TRUE TRUE _ TRUE _ _ TRUE _ _ TRUE TRUE TRUE _ TRUE _ _ _ _ _ TRUE _ _ TRUE _ _ TRUE TRUE _ _ _ _ TRUE w729 TRUE ("Yes") TRUE _ _ _ _] -> w151
          tunnel: w150 -> [_ _ _ _ _ _ _ _ w294 _ _ _ _ _ _ _ _ _ _ _ _ _ _ _ _ _ _ _ _ _ _ _ _ _ _ _ _ _ _ _ _ _ _ _ _ _ _ _ _ _ _]
          tunnel: w149 -> [_ _ w192 _ _ _ _ _ _ _ _ _ _ _ _ _ _ _ _ _ _ _ _ _ _ _ _ _ _ _ _ _ _ _ _ _ _ _ _ _ _ _ _ _ _ _ _ _ _ _ _]
          tunnel: w148 -> [w176 w185 w191 w214 w233 w242 w266 w276 w293 w309 w315 w326 w345 w353 w363 w368 w379 w391 w405 w422 w441 w448 w454 w472 w489 w504 w524 w542 w556 w561 w570 w588 w599 w602 w609 w626 w635 w646 w668 w673 w683 w692 w704 w721 w731 w740 w762 w784 w788 w791 w798]
          tunnel: [w172 w185 w190 w212 w232 w247 w259 w279 w292 w307 w314 w323 w344 w351 w361 w369 w378 w395 w404 w418 w435 w447 w452 w470 w488 w503 w517 w538 w556 w559 w568 w587 w599 w603 w614 w625 w634 w640 w663 w672 w685 w692 w696 w707 w731 w733 w759 w783 w788 w791 w798] -> w147
          tunnel: [_ _ _ _ _ _ _ _ _ _ _ w320 _ _ _ _ _ _ _ _ _ _ _ _ _ _ _ _ _ _ _ _ _ _ _ _ _ _ _ _ _ _ _ _ _ _ _ _ _ _ _] -> _
          tunnel: w145 -> [_ _ _ _ _ _ _ _ _ _ _ _ _ _ _ _ _ _ _ _ _ _ _ _ _ _ _ _ _ _ _ _ _ _ _ _ _ _ _ _ _ _ _ _ _ _ _ _ _ w792 w799]
          event "OK": Value Change {
            n86 = event-data() -> ()  [unwired: 2 out]
            n87 = call <resource>:"Finalize Text.vi"("error in (no error)"=w179, "Data in"=w176) -> ("error out"=w180:errorcluster, "Data out"=w175:T28)  [unwired: 8 out]
            n88 = call <resource>:"Finalize Movement.vi"("error in (no error)"=w180, "Data in"=w175) -> ("error out"=w181:errorcluster, "Data out"=w174:T28)  [unwired: 1 in, 7 out]
            n89 = call <resource>:"DeselectLayer.vi"("error in (no error)"=w181, "Data in"=w174) -> ("error out"=w178:errorcluster, "Data out"=w173:T28)  [unwired: 8 out]
            n90 = call <resource>:"Reset layer template selection.vi"("error in (no error)"=w178, "Data in"=w173) -> ("error out"=w177:errorcluster, "Data out"=w172:T28)  [unwired: 1 in, 7 out]
          }
          event "Cancel": Value Change {
            w186 = FALSE ("Yes")
            n91 = event-data() -> ()  [unwired: 2 out]
          }
          event Menu Selection (User); Menu Selection (App) {
            n92 = event-data() -> ("Type"=w196:T34, "ItemTag"=w197:string)  [unwired: 1 out]
            n93 = case shown="\"Text\"" w189 {
              tunnel: w195 -> [w198 w203]
              tunnel: w191 -> [w199 w202]
              tunnel: [w198 w201] -> w187
              tunnel: [w199 w200] -> w188
              frame Default {
              }
              frame "Text" {
                n94 = call <resource>:"Finalize Text.vi"("error in (no error)"=w203, "Data in"=w202) -> ("error out"=w201:errorcluster, "Data out"=w200:T28)  [unwired: 8 out]
              }
            }
            n95 = case shown="\"Menu Selection (User)\"" w196 {
              tunnel: w197 -> [_ w211]
              tunnel: [w205 w210] -> w193
              tunnel: w187 -> [w205 w209]
              tunnel: w192 -> [_ w208]
              tunnel: w188 -> [w204 w207]
              tunnel: [w204 w206] -> w190
              frame Default {
              }
              frame "Menu Selection (User)" {
                n96 = call <resource>:"MenuSelection(User).vi"("User events"=w208, "error in"=w209, "ItemTag"=w211, "Data in"=w207) -> ("error out"=w210:errorcluster, "Data out"=w206:T28)  [unwired: 1 in, 5 out]
              }
            }
          }
          event Mouse Down {
            n97 = event-data() -> ("CtlRef"=w217:refnum<vi>, "Button"=w213:u16)  [unwired: 1 out]
            n98 = case shown="1, 2" w213 {
              tunnel: w218 -> [w220 w227]
              tunnel: w217 -> [_ w231]
              tunnel: [w220 w225] -> w216
              tunnel: w214 -> [w219 w222]
              tunnel: [w219 w221] -> w212
              frame 0, Default {
              }
              frame 1, 2 {
                n99 = control-ref of="This VI"() -> (w230:refnum<vi>)
                n100 = call <resource>:"Defer_FP_Updates.vi"("Defer Panel Updates"=TRUE, "error in (no error)"=w227, "lv_icon.vi in"=w230) -> ("error out"=w228:errorcluster, "lv icon.vi out"=w223:refnum<vi>)  [unwired: 7 out]
                n101 = call <resource>:"Template_MouseDown.vi"("Add to Undo?"=TRUE, "error in"=w228, "CtlRef"=w231, "Data in"=w222) -> ("error out"=w226:errorcluster, "Data out"=w221:T28)  [unwired: 1 in, 5 out]
                n102 = call <resource>:"Defer_FP_Updates.vi"("error in (no error)"=w226, "lv_icon.vi in"=w223) -> ("error out"=w225:errorcluster)  [unwired: 1 in, 8 out]
              }
            }
          }
          event Value Change {
            n103 = event-data() -> ("NewVal"=w235:T21)  [unwired: 1 out]
            n104 = call <resource>:"Value Change_Tools.vi"("error in"=w236, "NewVal"=w235, "Data in"=w233) -> ("error out"=w234:errorcluster, "Data out"=w232:T28)  [unwired: 7 out]
          }
          event Mouse Down {
            n105 = event-data() -> ("Mods.Double Click"=w237:bool)  [unwired: 1 out]
            n106 = call <resource>:"Finalize Text.vi"("error in (no error)"=w243, "Data in"=w242) -> ("error out"=w245:errorcluster, "Data out"=w244:T28)  [unwired: 8 out]
            n107 = call <resource>:"Finalize Movement.vi"("error in (no error)"=w245, "Data in"=w244) -> ("error out"=w241:errorcluster, "Data out"=w240:T28)  [unwired: 1 in, 7 out]
            n108 = call <resource>:"Mouse Down.vi"("error in"=w241, "Double Click"=w237, "Data in"=w240) -> ("error out"=w238:errorcluster, "Data out"=w239:T28)  [unwired: 7 out]
            n109 = Bundle By Name(cluster=w239, "Support.Tool (old value)"=u32 111) -> (w247:T28)
          }
          event Value Change {
            # "Body Text Value Change event is fired programmatically during initialization so first call of this event is guaranteed to be a case we do not want to update the undo/redo information."
            n110 = event-data() -> ("OldVal"=w257:T8, "NewVal"=w256:T8, "OldVal.Body Text Spec.Alignment"=w261:T10)  [unwired: 1 out]
            n111 = Unbundle By Name(w257) -> ("Body Text Spec.Font"=w255:T9)
            n112 = Unbundle By Name(w256) -> ("Body Text Spec.Font"=w254:T9)
            n113 = local read "Tab Control"() -> (w252:T5)
            n114 = Unbundle By Name(w256) -> ("Body Text Spec.Alignment"=w262:T10)
            n115 = First Call?() -> (First Call?: T/F=w269:bool)
            n116 = Equal?(x=w252, y=T5."Icon Text") -> (x = y?=w250:bool)
            n117 = Not(x=w269) -> (.not. x?=w268:bool)
            n118 = Not Equal?(x=w255, y=w254) -> (x != y?=w253:bool)
            n119 = call <resource>:"Value Change_Body Text.vi"("Layer Icon"="Icon Text", "Add to Undo?"=w268, "error in"=w270, "NewVal"=w256, "Data in"=w266) -> ("error out"=w264:errorcluster, "Data out"=w263:T28)  [unwired: 5 out]
            n120 = And(x=w250, y=w253) -> (x .and. y?=w249:bool)
            n121 = Not Equal?(x=w262, y=w261) -> (x != y?=w260:bool)
            n122 = case shown="True" w249 {
              frame False {
              }
              frame True {
                n123 = property on="Line 1 text" class="Str"("Key Focus"=TRUE) -> ()  [unwired: 2 in, 2 out]
              }
            }
            n124 = call <resource>:"Alignment Value Change.vi"("Set Focus?"=w260, "error in"=w264, "NewVal"=w262, "Data in"=w263) -> ("error out"=w258:errorcluster, "Data out"=w259:T28)  [unwired: 6 out]
          }
          event Value Change {
            n125 = event-data() -> ()  [unwired: 2 out]
            n126 = call <resource>:"Finalize Text.vi"("error in (no error)"=w274, "Data in"=w276) -> ("error out"=w278:errorcluster, "Data out"=w277:T28)  [unwired: 8 out]
            n127 = local read "Line Color"() -> (w273:T20)
            n128 = local read "Fill Color"() -> (w283:T20)
            n129 = call <resource>:"Finalize Movement.vi"("error in (no error)"=w278, "Data in"=w277) -> ("error out"=w272:errorcluster, "Data out"=w275:T28)  [unwired: 1 in, 7 out]
            n130 = stacked-sequence {
              tunnel: w283 -> [w287]
              tunnel: [w286] -> w281
              tunnel: w273 -> [w285]
              tunnel: w272 -> [w284]
              frame #0 {
                n131 = local write "Fill Color"(w285) -> ()
                n132 = property on="Line Color" class="ColBox (strict)"(error in=w284, "Val(Sgnl)"=w287) -> (error out=w286:errorcluster)  [unwired: 1 in, 1 out]
              }
            }
            n133 = call <resource>:"Escape.vi"("error in"=w281, "Data in"=w275) -> ("error out"=w280:errorcluster, "Data out"=w279:T28)  [unwired: 1 in, 7 out]
          }
          event "Preview", "Terminals", "Preview2": Mouse Move {
            n134 = event-data() -> ("Coords"=w291:T31)  [unwired: 1 out]
            n135 = call <resource>:"CoordinatesCorrection.vi"("Coordinates In"=w291) -> ("Corrected Out"=w288:T31)  [unwired: 10 out]
            n136 = feedback-in #1(w288) -> ()
            n137 = feedback #1() -> (w290:T31)
            n138 = Not Equal?(x=w290, y=w288) -> (x != y?=w289:bool)
            n139 = case shown="True" w289 {
              tunnel: w297 -> [w299 w305]
              tunnel: [w299 w304] -> w296
              tunnel: w294 -> [_ w303]
              tunnel: w293 -> [w298 w302]
              tunnel: [w298 w301] -> w292
              tunnel: w288 -> [_ w300]
              frame False {
              }
              frame True {
                n140 = call <resource>:"MouseMove.vi"("Buffer"=w303, "error in"=w305, "Coords"=w300, "Data in"=w302) -> ("error out"=w304:errorcluster, "Data out"=w301:T28)  [unwired: 6 out]
              }
            }
          }
          event "Preview", "Terminals", "Preview2": Mouse Enter {
            n141 = event-data() -> ()  [unwired: 2 out]
            n142 = call <resource>:"SetCursor.vi"("error in (no error)"=w313, "Radio Buttons"=w311, "Data in"=w309) -> ("error out"=w312:errorcluster, "Data out"=w308:T28)  [unwired: 7 out]
            n143 = Bundle By Name(cluster=w308, "Support.Mouse inside icon?"=TRUE) -> (w307:T28)
          }
          event "Preview", "Terminals", "Preview2": Mouse Up {
            n144 = event-data() -> ("Coords"=w318:T31)  [unwired: 1 out]
            n145 = call <resource>:"PictureControl_MouseUp.vi"("error in"=w319, "Coords"=w318, "Data in"=w315) -> ("error out"=w316:errorcluster, "Data out"=w314:T28)  [unwired: 4 in, 3 out]
          }
          event Key Down?; event type 5.0.x8000000b {
            n146 = event-data() -> ("Type"=w325:T34, "Char"=w322:i16, "VKey"=w329:T35, "PlatMods"=w324:T36)  [unwired: 1 out]
            n147 = Equal?(x=i16 99, y=w322) -> (x = y?=w320:bool)
            n148 = call <resource>:"KeyDown.vi"("PlatMods"=w324, "Type"=w325, "error in (no error)"=w331, "VKey"=w329, "Char"=w322, "Data in"=w326) -> ("error out"=w330:errorcluster, "Discard?"=w328:bool, "Data out"=w323:T28)  [unwired: 3 out]
            n149 = event-data("Discard?"=w328) -> ()  [unwired: 1 in, 1 out]
          }
          event "Preview", "Terminals", "Preview2": Mouse Down {
            # "Left click"
            n150 = event-data() -> ("Button"=w334:u16, "Coords"=w347:T31)  [unwired: 1 out]
            n151 = Not Equal?(x=u16 1, y=w334) -> (x != y?=w332:bool)
            n152 = control-ref of="This VI"() -> (w343:refnum<vi>)
            n153 = call <resource>:"Defer_FP_Updates.vi"("Defer Panel Updates"=TRUE, "error in (no error)"=w349, "lv_icon.vi in"=w343) -> ("error out"=w339:errorcluster, "lv icon.vi out"=w341:refnum<vi>)  [unwired: 7 out]
            n154 = call <resource>:"Reset layer template selection.vi"("Force reset? (T)"=FALSE, "error in (no error)"=w339, "Data in"=w345) -> ("error out"=w338:errorcluster, "Data out"=w335:T28)  [unwired: 1 in, 6 out]
            n155 = call <resource>:"MouseDown.vi"("Flip colors?"=w332, "error in"=w338, "Coords"=w347, "Data in"=w335) -> ("error out"=w337:errorcluster, "Data out"=w344:T28)  [unwired: 1 in, 5 out]
            n156 = call <resource>:"Defer_FP_Updates.vi"("Defer Panel Updates"=FALSE, "error in (no error)"=w337, "lv_icon.vi in"=w341) -> ("error out"=w348:errorcluster)  [unwired: 8 out]
          }
          event Value Change {
            n157 = event-data() -> ()  [unwired: 2 out]
            n158 = call <vilib>:"Check Color.vi"("Color in"="Fill Color") -> ("Color out"=w356:T20)  [unwired: 26 out]
            n159 = call <vilib>:"Check Color.vi"("Color in"="Line Color") -> ("Color out"=w357:T20)  [unwired: 26 out]
            n160 = Bundle By Name(cluster=w353, "Support.Fill Color"=w356, "Support.Edge Color"=w357) -> (w352:T28)
            n161 = call <resource>:"Escape.vi"("Reset cursor (T)"=FALSE ("Reset cursor? (T)"), "error in"=w354, "Data in"=w352) -> ("error out"=w355:errorcluster, "Data out"=w351:T28)  [unwired: 1 in, 6 out]
          }
          event Key Up {
            n162 = event-data() -> ("PlatMods"=w362:T36)  [unwired: 1 out]
            n163 = call <resource>:"KeyUp.vi"("error in (no error)"=w364, "PlatMods"=w362, "Data in"=w363) -> ("error out"=w365:errorcluster, "Data out"=w361:T28)  [unwired: 7 out]
          }
          event Value Change {
            n164 = event-data() -> ()  [unwired: 2 out]
            n165 = call <resource>:"Finalize Text.vi"("error in (no error)"=w375, "Data in"=w368) -> ("error out"=w374:errorcluster, "Data out"=w370:T28)  [unwired: 8 out]
            n166 = call <resource>:"Finalize Movement.vi"("error in (no error)"=w374, "Data in"=w370) -> ("error out"=w371:errorcluster, "Data out"=w367:T28)  [unwired: 1 in, 7 out]
            n167 = call <resource>:"RotateFlip.vi"("error in"=w371, "Rotate"="Clockwise Rotate", "Data in"=w367) -> ("error out"=w372:errorcluster, "Data out"=w366:T28)  [unwired: 2 in, 5 out]
            n168 = call <resource>:"Escape.vi"("error in"=w372, "Data in"=w366) -> ("error out"=w373:errorcluster, "Data out"=w369:T28)  [unwired: 1 in, 7 out]
          }
          event Value Change {
            n169 = event-data() -> ("NewVal"=w388:variant)  [unwired: 1 out]
            n170 = control-ref of="This VI"() -> (w385:refnum<vi>)
            n171 = call <resource>:"Defer_FP_Updates.vi"("Defer Panel Updates"=TRUE, "error in (no error)"=w386, "lv_icon.vi in"=w385) -> ("error out"=w387:errorcluster, "lv icon.vi out"=w380:refnum<vi>)  [unwired: 7 out]
            n172 = call <resource>:"Mouse Down_Templates.vi"("Tag"="Templates", "error in"=w387, "NewVal"=w388, "Data in"=w379) -> ("error out"=w382:errorcluster, "Data out"=w378:T28)  [unwired: 1 in, 5 out]
            n173 = call <resource>:"Defer_FP_Updates.vi"("error in (no error)"=w382, "lv_icon.vi in"=w380) -> ("error out"=w383:errorcluster)  [unwired: 1 in, 8 out]
          }
          event User Event {
            # "This is an initialization event for the glyphs."
            n174 = event-data() -> ("Glyphs"=w403:string)  [unwired: 1 out]
            n175 = Unbundle By Name(w391) -> ("Ref.GlyphLoadAnimation"=w390:refnum<vi>, "Ref.refreshGlyphs"=w389:refnum<vi>)
            n176 = Unflatten From String(type="?", binary string=w403, error in (no error)=w401) -> (value=w398:T3[], error out=w400:errorcluster)  [unwired: 3 out]
            n177 = call <resource>:"Populate Graphics.vi"("error in"=w400, "Glyphs []"=w398, "Data in"=w391) -> ("error out"=w399:errorcluster, "Data out"=w395:T28)  [unwired: 7 out]
            n178 = call <resource>:"Write Glyphs to  File.vi"("File Name"="Glyphs.bin", "Path"=Pathes."Glyphs", "error in (no error)"=w399, "Graphics []"=w398) -> ("error out"=w394:errorcluster)  [unwired: 7 out]
            n179 = call <resource>:"ChangeRefreshGraphicsState.vi"("error in (no error)"=w394, "refreshing?"=FALSE, "button ref"=w389, "animatedDecoration ref"=w390) -> ("error out"=w393:errorcluster)  [unwired: 7 in]
          }
          event Mouse Down {
            n180 = event-data() -> ("PlatMods.Shift"=w406:bool, "CtlRef"=w416:refnum<vi>, "PlatMods.Ctrl"=w415:bool)  [unwired: 1 out]
            n181 = control-ref of="This VI"() -> (w412:refnum<vi>)
            n182 = call <resource>:"Defer_FP_Updates.vi"("Defer Panel Updates"=TRUE, "error in (no error)"=w413, "lv_icon.vi in"=w412) -> ("error out"=w411:errorcluster, "lv icon.vi out"=w408:refnum<vi>)  [unwired: 7 out]
            n183 = call <resource>:"Mouse Down_User Layers.vi"("Shift"=w406, "error in"=w411, "Ctrl"=w415, "CtlRef"=w416, "Data in"=w405) -> ("error out"=w410:errorcluster, "Data out"=w404:T28)  [unwired: 5 out]
            n184 = call <resource>:"Defer_FP_Updates.vi"("error in (no error)"=w410, "lv_icon.vi in"=w408) -> ("error out"=w409:errorcluster)  [unwired: 1 in, 8 out]
          }
          event "Filter glyphs by keyword": Mouse Down {
            # "If a mouse down event should\nselect the entered text, enable this case"
            n185 = event-data() -> ("CtlRef"=w425:refnum<vi>)  [unwired: 1 out]
            n186 = disable-structure shown="Enabled" {
              disable-tunnel: w426 -> [w429 w432]
              disable-tunnel: w425 -> [w428 _]
              disable-tunnel: [w427 w432] -> w424
              frame Disabled {
                n187 = property class="Str"(reference=w428, error in=w429, "Text.Selection Start"=u32 0 ("Text.Selection:Start"), "Text.Selection End"=-1 ("Text.Selection:End")) -> (error out=w427:errorcluster)  [unwired: 1 out]
              }
              frame Enabled {
              }
            }
            n188 = call <resource>:"Finalize Text.vi"("error in (no error)"=w424, "Data in"=w422) -> ("error out"=w423:errorcluster, "Data out"=w421:T28)  [unwired: 8 out]
            n189 = call <resource>:"DeselectLayer.vi"("error in (no error)"=w423, "Data in"=w421) -> ("error out"=w420:errorcluster, "Data out"=w419:T28)  [unwired: 8 out]
            n190 = call <resource>:"Escape.vi"("error in"=w420, "Data in"=w419) -> ("error out"=w417:errorcluster, "Data out"=w418:T28)  [unwired: 1 in, 7 out]
          }
          event "Filter glyphs by keyword": Value Change {
            n191 = event-data() -> ("NewVal"=w446:string)  [unwired: 1 out]
            n192 = Unbundle By Name(w441) -> ("Class.Glyph"=w442:refnum<class "Glyph.lvclass">, "Ref.DNL_Glyphs []"=w439:refnum<vi>, "Ref.Glyphs tree"=w438:refnum<vi>)
            n193 = First Call?() -> (First Call?: T/F=w444:bool)
            n194 = Not(x=w444) -> (.not. x?=w445:bool)
            n195 = call <resource>:"SearchGlyphs.vi"("Glyphs tree"=w438, "DNL_Glyphs []"=w439, "Reset position? (F)"=w445, "error in (no error)"=w443, "Keyword"=w446, "Glyph in"=w442) -> ("error out"=w437:errorcluster, "Glyph out"=w440:refnum<class "Glyph.lvclass">)  [unwired: 4 out]
            n196 = Bundle By Name(cluster=w441, "Class.Glyph"=w440) -> (w434:T28)
            n197 = call <resource>:"Add Data to History.vi"("Add to Undo?"=TRUE, "error in"=w437, "Data in"=w434) -> ("error out"=w436:errorcluster, "Data out"=w435:T28)  [unwired: 7 out]
          }
          event Mouse Down {
            n198 = event-data() -> ()  [unwired: 2 out]
            n199 = call <resource>:"MouseDown_Body Text.vi"("error in"=w451, "Data in"=w448) -> ("error out"=w450:errorcluster, "Data out"=w447:T28)  [unwired: 8 out]
          }
          event Value Change {
            n200 = event-data() -> ("OldVal.Opacity"=w457:u8, "NewVal.Opacity"=w456:u8, "NewVal"=w462:T15)  [unwired: 1 out]
            n201 = Not Equal?(x=w457, y=w456) -> (x != y?=w455:bool)
            n202 = call <resource>:"Value Change_Top or Bottom Layer.vi"("Type"=enum16{"Template Layer", "Text Layer"}."Text Layer", "error in (no error)"=w463, "Data"=w462, "Data in"=w454) -> ("error out"=w459:errorcluster, "Data out"=w453:T28)  [unwired: 6 out]
            n203 = case shown="True" w455 {
              tunnel: w459 -> [w465 w469]
              tunnel: [w465 w468] -> w458
              tunnel: w453 -> [w464 w467]
              tunnel: [w464 w466] -> w452
              frame False {
              }
              frame True {
                n204 = call <resource>:"Reset layer template selection.vi"("error in (no error)"=w469, "Data in"=w467) -> ("error out"=w468:errorcluster, "Data out"=w466:T28)  [unwired: 1 in, 7 out]
              }
            }
          }
          event Value Change {
            n205 = event-data() -> ("OldVal.Opacity"=w474:u8, "NewVal.Opacity"=w475:u8, "NewVal"=w479:T15)  [unwired: 1 out]
            n206 = Not Equal?(x=w474, y=w475) -> (x != y?=w473:bool)
            n207 = call <resource>:"Value Change_Top or Bottom Layer.vi"("Type"=enum16{"Template Layer", "Text Layer"}."Template Layer", "error in (no error)"=w481, "Data"=w479, "Data in"=w472) -> ("error out"=w477:errorcluster, "Data out"=w471:T28)  [unwired: 6 out]
            n208 = case shown="False" w473 {
              tunnel: w477 -> [w483 w487]
              tunnel: [w483 w486] -> w476
              tunnel: w471 -> [w482 w485]
              tunnel: [w482 w484] -> w470
              frame False {
              }
              frame True {
                n209 = call <resource>:"Reset layer template selection.vi"("error in (no error)"=w487, "Data in"=w485) -> ("error out"=w486:errorcluster, "Data out"=w484:T28)  [unwired: 1 in, 7 out]
              }
            }
          }
          event Value Change {
            n210 = event-data() -> ("NewVal"=w498:variant)  [unwired: 1 out]
            n211 = control-ref of="This VI"() -> (w495:refnum<vi>)
            n212 = call <resource>:"Defer_FP_Updates.vi"("Defer Panel Updates"=TRUE, "error in (no error)"=w494, "lv_icon.vi in"=w495) -> ("error out"=w493:errorcluster, "lv icon.vi out"=w490:refnum<vi>)  [unwired: 7 out]
            n213 = Variant To Data(error in=w493, type=0, Variant=w498) -> (data=w497:i32, error out=w499:errorcluster)
            n214 = call <resource>:"UpdateLayerView_ScrollbarChanged.vi"("error in"=w499, "Scrollbar Position"=w497, "Data in"=w489) -> ("error out"=w492:errorcluster, "Data out"=w488:T28)  [unwired: 7 out]
            n215 = call <resource>:"Defer_FP_Updates.vi"("error in (no error)"=w492, "lv_icon.vi in"=w490) -> ("error out"=w491:errorcluster)  [unwired: 1 in, 8 out]
          }
          event Value Change {
            # "We do not use the dynamic registerd event for Layer Clust.Value Change\nbecause it would be a huge effort to lock the front panel until this\nevent case has been completed."
            n216 = event-data() -> ("OldVal.Visibility?"=w502:bool, "CtlRef"=w516:refnum<vi>, "OldVal.LayerName"=w501:string)  [unwired: 1 out]
            n217 = control-ref of="This VI"() -> (w513:refnum<vi>)
            n218 = call <resource>:"Defer_FP_Updates.vi"("Defer Panel Updates"=TRUE, "error in (no error)"=w512, "lv_icon.vi in"=w513) -> ("error out"=w511:errorcluster, "lv icon.vi out"=w508:refnum<vi>)  [unwired: 7 out]
            n219 = call <resource>:"LayerCluster_ValueChange.vi"("Old Visibility?"=w502, "error in"=w511, "Old name"=w501, "CtlRef"=w516, "Data in"=w504) -> ("error out"=w510:errorcluster, "Data out"=w505:T28)  [unwired: 1 in, 4 out]
            n220 = call <resource>:"Defer_FP_Updates.vi"("Defer Panel Updates"=FALSE, "error in (no error)"=w510, "lv_icon.vi in"=w508) -> ("error out"=w507:errorcluster)  [unwired: 8 out]
            n221 = call <resource>:"Reset layer template selection.vi"("error in (no error)"=w507, "Data in"=w505) -> ("error out"=w506:errorcluster, "Data out"=w503:T28)  [unwired: 1 in, 7 out]
          }
          event "Filter templates by keyword": Value Change {
            n222 = event-data() -> ("NewVal"=w536:string)  [unwired: 1 out]
            n223 = Unbundle By Name(w524) -> ("Ref.Templates tree"=w522:refnum<vi>, "Class.Templates"=w525:refnum<class "FakedArray.lvclass">)
            n224 = control-ref of="This VI"() -> (w535:refnum<vi>)
            n225 = call <resource>:"Defer_FP_Updates.vi"("Defer Panel Updates"=TRUE, "error in (no error)"=w533, "lv_icon.vi in"=w535) -> ("error out"=w527:errorcluster, "lv icon.vi out"=w532:refnum<vi>)  [unwired: 7 out]
            n226 = call-dynamic "SET_ScrollbarPosition.vi"("error in (no error)"=w527, "FakedArray.lvclass in"=w525) -> ("error out"=w528:errorcluster, "FakedArray.lvclass out"=w529:refnum<class "FakedArray.lvclass">)  [unwired: 1 in, 7 out]
            n227 = call <resource>:"ResetColor.vi"("error in (no error)"=w528, "FakedArray in"=w529) -> ("error out"=w530:errorcluster, "FakedArray out"=w531:refnum<class "FakedArray.lvclass">)  [unwired: 8 out]
            n228 = call-dynamic "UpdateVisibleData.vi"("Templates tree"=w522, "error in (no error)"=w530, "Keyword"=w536, "FakedArray in"=w531) -> ("error out"=w526:errorcluster, "FakedArray out"=w523:refnum<class "FakedArray.lvclass">)  [unwired: 1 in, 5 out]
            n229 = Bundle By Name(cluster=w524, "Class.Templates"=w523) -> (w518:T28)
            n230 = call <resource>:"Defer_FP_Updates.vi"("error in (no error)"=w526, "lv_icon.vi in"=w532) -> ("error out"=w520:errorcluster)  [unwired: 1 in, 8 out]
            n231 = call <resource>:"Add Data to History.vi"("Add to Undo?"=TRUE, "error in"=w520, "Data in"=w518) -> ("error out"=w519:errorcluster, "Data out"=w517:T28)  [unwired: 7 out]
          }
          event "Filter templates by keyword": Mouse Down {
            # "If a mouse down event should\nselect the entered text, enable this case"
            n232 = event-data() -> ("CtlRef"=w546:refnum<vi>)  [unwired: 1 out]
            n233 = disable-structure shown="Enabled" {
              disable-tunnel: w546 -> [w551 _]
              disable-tunnel: w545 -> [w549 w552]
              disable-tunnel: [w547 w552] -> w544
              frame Disabled {
                n234 = property class="Str"(reference=w551, error in=w549, "Text.Selection Start"=u32 0 ("Text.Selection:Start"), "Text.Selection End"=-1 ("Text.Selection:End")) -> (error out=w547:errorcluster)  [unwired: 1 out]
              }
              frame Enabled {
              }
            }
            n235 = call <resource>:"Finalize Text.vi"("error in (no error)"=w544, "Data in"=w542) -> ("error out"=w543:errorcluster, "Data out"=w541:T28)  [unwired: 8 out]
            n236 = call <resource>:"DeselectLayer.vi"("error in (no error)"=w543, "Data in"=w541) -> ("error out"=w540:errorcluster, "Data out"=w539:T28)  [unwired: 8 out]
            n237 = call <resource>:"Escape.vi"("error in"=w540, "Data in"=w539) -> ("error out"=w537:errorcluster, "Data out"=w538:T28)  [unwired: 1 in, 7 out]
          }
          event "Help": Value Change {
            n238 = event-data() -> ()  [unwired: 2 out]
            n239 = control-ref of="This VI"() -> (w555:refnum<vi>)
            n240 = property class="VI"(reference=w555) -> (error out=w553:errorcluster, "Help.URL"=w554:string)  [unwired: 1 in, 1 out]
            n241 = call <resource>:"IE_Open Help Link.vi"("error in (no error)"=w553, "Help.URL"=w554) -> ()  [unwired: 9 in, 1 out]
          }
          event "Glyphs": Value Change {
            n242 = event-data() -> ("NewVal"=w565:string)  [unwired: 1 out]
            n243 = Unbundle By Name(w561) -> ("Class.Glyph"=w562:refnum<class "Glyph.lvclass">, "Ref.DNL_Glyphs []"=w558:refnum<vi>)
            n244 = call <resource>:"FilterGlyphs.vi"("error in (no error)"=w563, "DNL_Glyphs []"=w558, "Tag"=w565, "Glyph in"=w562) -> ("error out"=w564:errorcluster, "Glyph out"=w560:refnum<class "Glyph.lvclass">)  [unwired: 6 out]
            n245 = Bundle By Name(cluster=w561, "Class.Glyph"=w560) -> (w559:T28)
          }
          event "Templates": Value Change {
            n246 = event-data() -> ("CtlRef"=w567:refnum<vi>, "NewVal"=w579:string)  [unwired: 1 out]
            n247 = control-ref of="This VI"() -> (w583:refnum<vi>)
            n248 = Unbundle By Name(w570) -> ("Class.Templates"=w571:refnum<class "FakedArray.lvclass">)
            n249 = call <resource>:"Defer_FP_Updates.vi"("Defer Panel Updates"=TRUE, "error in (no error)"=w581, "lv_icon.vi in"=w583) -> ("error out"=w573:errorcluster, "lv icon.vi out"=w578:refnum<vi>)  [unwired: 7 out]
            n250 = call-dynamic "SET_ScrollbarPosition.vi"("error in (no error)"=w573, "FakedArray.lvclass in"=w571) -> ("error out"=w575:errorcluster, "FakedArray.lvclass out"=w574:refnum<class "FakedArray.lvclass">)  [unwired: 1 in, 7 out]
            n251 = local write "Filter templates by keyword"("") -> ()
            n252 = call <resource>:"ResetColor.vi"("error in (no error)"=w575, "FakedArray in"=w574) -> ("error out"=w576:errorcluster, "FakedArray out"=w577:refnum<class "FakedArray.lvclass">)  [unwired: 8 out]
            n253 = call-dynamic "UpdateVisibleData.vi"("Templates tree"=w567, "error in (no error)"=w576, "Tag"=w579, "FakedArray in"=w577) -> ("error out"=w572:errorcluster, "FakedArray out"=w569:refnum<class "FakedArray.lvclass">)  [unwired: 1 in, 5 out]
            n254 = Bundle By Name(cluster=w570, "Class.Templates"=w569) -> (w568:T28)
            n255 = call <resource>:"Defer_FP_Updates.vi"("error in (no error)"=w572, "lv_icon.vi in"=w578) -> ("error out"=w580:errorcluster)  [unwired: 1 in, 8 out]
          }
          event Value Change {
            n256 = event-data() -> ()  [unwired: 2 out]
            n257 = control-ref of="This VI"() -> (w594:refnum<vi>)
            n258 = call <resource>:"Defer_FP_Updates.vi"("Defer Panel Updates"=TRUE, "error in (no error)"=w593, "lv_icon.vi in"=w594) -> ("error out"=w592:errorcluster, "lv icon.vi out"=w591:refnum<vi>)  [unwired: 7 out]
            n259 = call <resource>:"MoveLayers.vi"("error in"=w592, "Arrow Up"="Move Up", "Data in"=w588) -> ("error out"=w584:errorcluster, "Data out"=w587:T28)  [unwired: 7 out]
            n260 = stacked-sequence {
              tunnel: [w597] -> w585
              tunnel: w584 -> [w597]
              frame #0 {
                w598 = FALSE ("Arrow Down")
                n261 = local write "Move Down"(w598) -> ()
                n262 = local write "Move Up"(w598) -> ()
              }
            }
            n263 = call <resource>:"Defer_FP_Updates.vi"("Defer Panel Updates"=FALSE, "error in (no error)"=w585, "lv_icon.vi in"=w591) -> ("error out"=w590:errorcluster)  [unwired: 8 out]
          }
          event Shortcut Menu Activation? {
            n264 = event-data() -> ()  [unwired: 2 out]
            n265 = event-data("Discard?"=TRUE) -> ()  [unwired: 1 in, 1 out]
          }
          event Mouse Leave; Mouse Up {
            n266 = event-data() -> ()  [unwired: 2 out]
            n267 = call <resource>:"Add Data to History.vi"("Add to Undo?"=TRUE, "error in"=w605, "Data in"=w602) -> ("error out"=w604:errorcluster, "Data out"=w603:T28)  [unwired: 7 out]
          }
          event User Event {
            # "This is an initialization event for the templates"
            n268 = event-data() -> ("Templates"=w624:string)  [unwired: 1 out]
            n269 = Unbundle By Name(w609) -> ("Ref.TemplateLoadAnimation"=w608:refnum<vi>, "Ref.refreshTemplates"=w607:refnum<vi>)
            n270 = control-ref of="This VI"() -> (w619:refnum<vi>)
            n271 = call <resource>:"Defer_FP_Updates.vi"("Defer Panel Updates"=TRUE, "error in (no error)"=w622, "lv_icon.vi in"=w619) -> ("error out"=w617:errorcluster, "lv icon.vi out"=w616:refnum<vi>)  [unwired: 7 out]
            n272 = Unflatten From String(type="?", binary string=w624, error in (no error)=w617) -> (value=w615:cluster{T1[], i32, bool}, error out=w620:errorcluster)  [unwired: 3 out]
            n273 = call <resource>:"Process Template Graphics.vi"("error in (no error)"=w620, "Data"=w615, "Data in"=w609) -> ("error out"=w612:errorcluster, "Data out"=w614:T28)  [unwired: 7 out]
            n274 = call <resource>:"ChangeRefreshGraphicsState.vi"("error in (no error)"=w612, "refreshing?"=FALSE, "button ref"=w607, "animatedDecoration ref"=w608) -> ("error out"=w611:errorcluster)  [unwired: 7 in]
            n275 = call <resource>:"Defer_FP_Updates.vi"("error in (no error)"=w611, "lv_icon.vi in"=w616) -> ("error out"=w613:errorcluster)  [unwired: 1 in, 8 out]
          }
          event "Templates": Mouse Down {
            n276 = event-data() -> ("CtlRef"=w629:refnum<vi>, "Coords"=w631:T31)  [unwired: 1 out]
            n277 = call <resource>:"Mouse Down_Tree.vi"("Tree"=w629, "error in (no error)"=w630, "Coords"=w631) -> ("error out"=w628:errorcluster)  [unwired: 8 out]
            n278 = call <resource>:"Escape.vi"("error in"=w628, "Data in"=w626) -> ("error out"=w627:errorcluster, "Data out"=w625:T28)  [unwired: 1 in, 7 out]
          }
          event "Glyphs": Mouse Down {
            n279 = event-data() -> ("CtlRef"=w633:refnum<vi>, "Coords"=w638:T31)  [unwired: 1 out]
            n280 = local write "Filter glyphs by keyword"("") -> ()
            n281 = call <resource>:"Mouse Down_Tree.vi"("Tree"=w633, "error in (no error)"=w639, "Coords"=w638) -> ("error out"=w637:errorcluster)  [unwired: 8 out]
            n282 = call <resource>:"Escape.vi"("error in"=w637, "Data in"=w635) -> ("error out"=w636:errorcluster, "Data out"=w634:T28)  [unwired: 1 in, 7 out]
          }
          event "Tab Control": Value Change {
            n283 = event-data() -> ("NewVal"=w651:T5)  [unwired: 1 out]
            n284 = case shown="\"Templates\"" w651 {
              tunnel: w650 -> [w655 w658 w660 w662]
              tunnel: [w654 w657 w661 w662] -> w649
              frame "Templates" {
                n285 = property on="Filter templates by keyword" class="Str"(error in=w655, "Key Focus"=TRUE) -> (error out=w654:errorcluster)  [unwired: 1 in, 1 out]
              }
              frame "Glyphs" {
                n286 = property on="Filter glyphs by keyword" class="Str"(error in=w658, "Key Focus"=TRUE) -> (error out=w657:errorcluster)  [unwired: 1 in, 1 out]
              }
              frame "Icon Text" {
                n287 = property on="Line 1 text" class="Str"(error in=w660, "Key Focus"=TRUE) -> (error out=w661:errorcluster)  [unwired: 1 in, 1 out]
              }
              frame "Layers", Default {
              }
            }
            n288 = call <resource>:"Finalize Text.vi"("error in (no error)"=w649, "Data in"=w646) -> ("error out"=w652:errorcluster, "Data out"=w645:T28)  [unwired: 8 out]
            n289 = call <resource>:"Finalize Movement.vi"("error in (no error)"=w652, "Data in"=w645) -> ("error out"=w644:errorcluster, "Data out"=w642:T28)  [unwired: 1 in, 7 out]
            n290 = call <resource>:"Escape.vi"("error in"=w644, "Data in"=w642) -> ("error out"=w643:errorcluster, "Data out"=w641:T28)  [unwired: 1 in, 7 out]
            n291 = call <resource>:"Reset layer template selection.vi"("error in (no error)"=w643, "Data in"=w641) -> ("error out"=w648:errorcluster, "Data out"=w640:T28)  [unwired: 1 in, 7 out]
          }
          event Mouse Down {
            n292 = event-data() -> ()  [unwired: 2 out]
            n293 = call <resource>:"Finalize Text.vi"("error in (no error)"=w669, "Data in"=w668) -> ("error out"=w670:errorcluster, "Data out"=w667:T28)  [unwired: 8 out]
            n294 = call <resource>:"Finalize Movement.vi"("error in (no error)"=w670, "Data in"=w667) -> ("error out"=w666:errorcluster, "Data out"=w664:T28)  [unwired: 1 in, 7 out]
            n295 = call <resource>:"Escape.vi"("error in"=w666, "Data in"=w664) -> ("error out"=w665:errorcluster, "Data out"=w663:T28)  [unwired: 1 in, 7 out]
          }
          event Mouse Down {
            n296 = event-data() -> ("Button"=w674:u16)  [unwired: 1 out]
            n297 = case shown="1" w674 {
              tunnel: w676 -> [w678 w682]
              tunnel: [w678 w681] -> w675
              tunnel: w673 -> [w677 w680]
              tunnel: [w677 w679] -> w672
              frame 0, Default {
              }
              frame 1 {
                # "Left click"
                n298 = call <resource>:"Reset layer template selection.vi"("error in (no error)"=w682, "Data in"=w680) -> ("error out"=w681:errorcluster, "Data out"=w679:T28)  [unwired: 1 in, 7 out]
              }
            }
          }
          event "Preview", "Preview2", "Terminals": Mouse Leave {
            n299 = event-data() -> ()  [unwired: 2 out]
            n300 = Bundle By Name(cluster=w683, "Support.Mouse inside icon?"=FALSE) -> (w685:T28)
          }
          event Mouse Down {
            n301 = event-data() -> ("CtlRef"=w691:refnum<vi>)  [unwired: 1 out]
            n302 = property class="CmbBox (strict)"(reference=w691, error in=w690, "Text.Selection Start"=u32 0 ("Text.Selection:Start"), "Text.Selection End"=u32 1000 ("Text.Selection:End")) -> (error out=w689:errorcluster)  [unwired: 1 out]
          }
          event Value Change {
            n303 = event-data() -> ()  [unwired: 2 out]
            n304 = control-ref of="This VI"() -> (w703:refnum<vi>)
            n305 = call <resource>:"Defer_FP_Updates.vi"("Defer Panel Updates"=TRUE, "error in (no error)"=w702, "lv_icon.vi in"=w703) -> ("error out"=w700:errorcluster, "lv icon.vi out"=w699:refnum<vi>)  [unwired: 7 out]
            n306 = call <resource>:"Add new Layer.vi"("error in"=w700, "Data in"=w704) -> ("error out"=w695:errorcluster, "Data out"=w697:T28)  [unwired: 8 out]
            n307 = call <resource>:"ViewLayer.vi"("Add to Undo?"=TRUE, "error in (no error)"=w695, "Data in"=w697) -> ("error out"=w694:errorcluster, "Data out"=w696:T28)  [unwired: 1 in, 6 out]
            n308 = call <resource>:"Defer_FP_Updates.vi"("error in (no error)"=w694, "lv_icon.vi in"=w699) -> ("error out"=w698:errorcluster)  [unwired: 1 in, 8 out]
          }
          event Value Change {
            n309 = event-data() -> ()  [unwired: 2 out]
            n310 = control-ref of="This VI"() -> (w715:refnum<vi>)
            n311 = Unbundle By Name(w721) -> ("Class.Icon"=w720:refnum<class "Icon.lvclass">)
            n312 = call <resource>:"Defer_FP_Updates.vi"("Defer Panel Updates"=TRUE, "error in (no error)"=w714, "lv_icon.vi in"=w715) -> ("error out"=w713:errorcluster, "lv icon.vi out"=w712:refnum<vi>)  [unwired: 7 out]
            n313 = call-dynamic "GET_All User Layers.vi"("error in (no error)"=w713, "Icon.lvclass in"=w720) -> ("error out"=w727:errorcluster, "User Layer"=w723:refnum<class "Layer.lvclass">[], "Icon.lvclass out"=w722:refnum<class "Icon.lvclass">)  [unwired: 7 out]
            n314 = call <resource>:"Delete Selected Layers.vi"("error in"=w727, "All Layers in"=w723, "Data in"=w721) -> ("error out"=w726:errorcluster, "All Layers out"=w724:refnum<class "Layer.lvclass">[], "Data out"=w718:T28)
            n315 = call-dynamic "SET_UserLayers.vi"("error in (no error)"=w726, "Layers"=w724, "Icon.lvclass in"=w722) -> ("error out"=w725:errorcluster, "Icon.lvclass out"=w719:refnum<class "Icon.lvclass">)  [unwired: 7 in]
            n316 = Bundle By Name(cluster=w718, "Class.Icon"=w719) -> (w717:T28)
            n317 = call <resource>:"Reset layer template selection.vi"("error in (no error)"=w725, "Data in"=w717) -> ("error out"=w706:errorcluster, "Data out"=w708:T28)  [unwired: 1 in, 7 out]
            n318 = call <resource>:"ViewLayer.vi"("Add to Undo?"=TRUE, "error in (no error)"=w706, "Data in"=w708) -> ("error out"=w705:errorcluster, "Data out"=w707:T28)  [unwired: 2 in, 5 out]
            n319 = call <resource>:"Defer_FP_Updates.vi"("error in (no error)"=w705, "lv_icon.vi in"=w712) -> ("error out"=w711:errorcluster)  [unwired: 1 in, 8 out]
          }
          event Panel Close? {
            w729 = FALSE ("Yes")
            n320 = event-data() -> ()  [unwired: 2 out]
            n321 = event-data("Discard?"=TRUE) -> ()  [unwired: 1 in, 1 out]
          }
          event Mouse Up {
            n322 = event-data() -> ()  [unwired: 2 out]
            n323 = Unbundle By Name(w740) -> ("Support.Action"=w738:T32, "Support.Mouse inside icon?"=w743:bool, "Support.Mouse Move Coords"=w739:T31)
            n324 = case shown="False" w743 {
              tunnel: w741 -> [w747 w758]
              tunnel: [w745 w758] -> w736
              tunnel: [w748 w757] -> w734
              tunnel: w740 -> [w749 w757]
              tunnel: w739 -> [w746 _]
              tunnel: w738 -> [w744 _]
              frame False {
                n325 = case shown="\"Move Selection\", \"Tool\"" w744 {
                  tunnel: w749 -> [w751 w756]
                  tunnel: [w751 w755] -> w748
                  tunnel: w747 -> [w750 w754]
                  tunnel: w746 -> [_ w753]
                  tunnel: [w750 w752] -> w745
                  frame "Default", Default {
                  }
                  frame "Move Selection", "Tool" {
                    n326 = call <resource>:"PictureControl_MouseUp.vi"("error in"=w754, "Coords"=w753, "Data in"=w756) -> ("error out"=w752:errorcluster, "Data out"=w755:T28)  [unwired: 4 in, 3 out]
                  }
                }
              }
              frame True {
              }
            }
            n327 = call <resource>:"Add Data to History.vi"("Check special fields? (F)"=TRUE, "Add to Undo?"=TRUE, "error in"=w736, "Data in"=w734) -> ("error out"=w735:errorcluster, "Data out"=w733:T28)  [unwired: 6 out]
          }
          event "Glyphs []": Mouse Down {
            n328 = event-data() -> ("Button"=w767:u16, "Mods.Double Click"=w768:bool, "CtlRef"=w770:refnum<vi>, "Coords"=w771:T31)  [unwired: 1 out]
            n329 = case shown="1" w767 {
              tunnel: w771 -> [_ w780]
              tunnel: w770 -> [_ w779]
              tunnel: [w773 w778] -> w764
              tunnel: w769 -> [w773 w777]
              tunnel: w768 -> [_ w776]
              tunnel: w762 -> [w772 w775]
              tunnel: [w772 w774] -> w760
              frame 0, Default {
              }
              frame 1 {
                # "Left click"
                n330 = call <resource>:"Mouse Down_Glyphs.vi"("Double Click"=w776, "Coords"=w780, "error in"=w777, "CtlRef"=w779, "Data in"=w775) -> ("error out"=w778:errorcluster, "Data out"=w774:T28)  [unwired: 1 in, 4 out]
              }
            }
            n331 = call <resource>:"Reset layer template selection.vi"("error in (no error)"=w764, "Data in"=w760) -> ("error out"=w763:errorcluster, "Data out"=w761:T28)  [unwired: 1 in, 7 out]
            n332 = call <resource>:"Update glyph path string.vi"("error in (no error)"=w763, "Data in"=w761) -> ("error out"=w765:errorcluster, "Data out"=w759:T28)  [unwired: 1 in, 7 out]
          }
          event Mouse Down {
            n333 = event-data() -> ()  [unwired: 2 out]
            n334 = call <resource>:"Escape.vi"("error in"=w782, "Data in"=w784) -> ("error out"=w781:errorcluster, "Data out"=w783:T28)  [unwired: 1 in, 7 out]
          }
          event "Glyphs", "Templates": Item Close; "Glyphs", "Templates": event #0x1e {
            n335 = event-data() -> ("CtlRef"=w785:refnum<vi>)  [unwired: 1 out]
            n336 = call <resource>:"DealWithScrollbars.vi"("error in (no error)"=w787, "Tree"=w785) -> ("error out"=w786:errorcluster)  [unwired: 9 in]
          }
          event Value Change {
            n337 = event-data() -> ()  [unwired: 2 out]
            n338 = Unbundle By Name(w791) -> ("Ref.GlyphLoadAnimation"=w789:refnum<vi>, "Ref.refreshGlyphs"=w790:refnum<vi>)
            n339 = call <resource>:"Launch Dynamically Load Graphics.vi"("User events"=w792, "Path"=Pathes."Glyphs", "error in (no error)"=w794, "button ref"=w790, "animatedDecoration ref"=w789) -> ("error out"=w793:errorcluster)  [unwired: 1 in, 5 out]
          }
          event Value Change {
            n340 = event-data() -> ()  [unwired: 2 out]
            n341 = Unbundle By Name(w798) -> ("Ref.TemplateLoadAnimation"=w796:refnum<vi>, "Ref.refreshTemplates"=w797:refnum<vi>)
            n342 = call <resource>:"Launch Dynamically Load Graphics.vi"("User events"=w799, "Path"=Pathes."Icon Templates", "error in (no error)"=w801, "button ref"=w797, "animatedDecoration ref"=w796) -> ("error out"=w800:errorcluster)  [unwired: 1 in, 5 out]
          }
        }
        n343 = case shown="True" w151 {
          tunnel: [_ w166] -> w155
          tunnel: w154 -> [w163 w169]
          tunnel: [w163 w168] -> w153
          tunnel: "Tools" -> [_ w167]
          tunnel: w147 -> [w162 w165]
          tunnel: [w162 w164] -> w146
          frame False {
          }
          frame True {
            n344 = call <resource>:"DrawIcon.vi"("Tools"=w167, "error in (no error)"=w169, "Data in"=w165) -> ("error out"=w168:errorcluster, "Icon"=w166:picture, "Data out"=w164:T28, "RGB"=→"RGB":string, "XYL"=→"XYZ":string)  [unwired: 2 in, 2 out]
            "Icon" <- w166
            "Preview" <- w166
          }
        }
        n345 = Unbundle By Name(w154) -> ("status"=w160:bool)
        n346 = Or(x=w160, y=w159) -> (x .or. y?=w158:bool)
      }
      n347 = call <resource>:"Buffer for lossless tracking.vi"("Ref Cluster"=w128, "User events"=w131, "error in (no error)"=w133, "Buffer"=w132) -> ()  [unwired: 8 out]
      n348 = call <resource>:"Extract LV Icon Data.vi"("error in (no error)"=w122, "LabVIEW Icon in (original)"=w120, "Data in"=w124) -> ("error out"=w121:errorcluster, "LabVIEW Icon out"=w123:string, "Data out"=w119:T28)  [unwired: 6 in]
      n349 = call <vilib>:"Get Image Data.vi"("Pic In"=w140) -> ("image data out"=w127:T4)  [unwired: 2 in, 8 out]
      n350 = call <vilib>:"Get Image Data.vi"("depth (24)"=1 ("depth"), "Pic In"=w140) -> ("image data out"=w138:T4)  [unwired: 2 in, 7 out]
      n351 = call <resource>:"SetCursor.vi"("Radio Buttons"=Tools."Select", "Data in"=w119) -> ("Data out"=w118:T28)  [unwired: 8 in, 1 out]
      n352 = Unbundle By Name(w121) -> ("code"=w141:i32)
      n353 = flat-sequence {
        tunnel: w144 -> [w817]
        tunnel: w142 -> [w814]
        tunnel: w121 -> [w813]
        tunnel: w131 -> [w811]
        tunnel: w118 -> [w807]
        tunnel: w115 -> [w805]
        tunnel: [w805] -> w114
        tunnel: [w804] -> w113
        tunnel: [w803] -> w112
        tunnel: w111 -> [w803]
        tunnel: w114 -> [w822]
        tunnel: w113 -> [w821]
        tunnel: w112 -> [w819]
        frame #0 {
          n354 = Unbundle By Name(w811) -> ("Global stop?"=w810:refnum<user-event>, "Templates"=w809:refnum<user-event>, "Glyphs"=w808:refnum<user-event>)
          n355 = Unbundle(w817) -> ("Events"=w816:refnum<event-registration>)
          n356 = call <resource>:"Write INI Tokens and VI Tags.vi"("error in (no error)"=w813, "Data in"=w807) -> ("error out"=w806:errorcluster)  [unwired: 1 in, 8 out]
          n357 = Unregister For Events(event registration refnum=w816) -> ()  [unwired: 1 in, 1 out]
          n358 = flat-sequence {
            tunnel: w806 -> [_]
            tunnel: [w818] -> w804
            frame #0 {
              n359 = call <resource>:"Call Keep IE in Memory.vi"() -> ()  [unwired: 1 out]
            }
            frame #1 {
              n360 = property class="VI"() -> ("Front Panel.WinBounds"=w818:T37)  [unwired: 2 in, 2 out]
            }
          }
          n361 = Release Notifier(notifier=w814, force destroy? (F)=TRUE) -> ()  [unwired: 1 in, 3 out]
          n362 = Generate User Event(user event=w810, event data cluster=TRUE) -> ()  [unwired: 2 in, 2 out]
          n363 = Destroy User Event(user event=w809) -> ()  [unwired: 1 in, 1 out]
          n364 = Destroy User Event(user event=w808) -> ()  [unwired: 1 in, 1 out]
        }
        frame #1 {
          n365 = Equal?(x=w821, y=w822) -> (x = y?=w820:bool)
          n366 = case shown="False" w820 {
            tunnel: w821 -> [w830 _]
            tunnel: w819 -> [w823 _]
            frame False {
              # "Bounds changed...write new bounds\nto INI file"
              n367 = Unbundle(w830) -> ("Left"=w829:i16, "Top"=w828:i16, "Right"=w827:i16, "Bottom"=w826:i16)
              n368 = Format Into String(format string="%d,%d,%d,%d", w829, w828, w827, w826) -> (resulting string=w824:string)  [unwired: 2 in, 1 out]
              n369 = call-by-ref "?"("value"=w824, "key"=w823) -> ()  [unwired: 3 in, 7 out]
            }
            frame True {
              # "Bounds didn't change while window was\nopen...don't do anything"
            }
          }
        }
        frame #2 {
          n370 = invoke class="VI" method="FP.Close"() -> ()  [unwired: 3 in, 3 out]
        }
      }
      n371 = call-dynamic "GET_Notifier.vi"("error in (no error)"=w125, "Ants.lvclass in"=w129) -> ("error out"=w136:errorcluster, "Notifier"=w142:refnum<notifier>, "Ants.lvclass out"=w137:refnum<class "Ants.lvclass">)  [unwired: 7 out]
      n372 = call <resource>:"RunningAnts.vi"("error in (no error)"=w136, "Ants in"=w137) -> ()  [unwired: 10 out]
    }
    frame Error {
      n373 = Unbundle By Name(w832) -> ("code"=w833:i32)
      n374 = call <vilib>:"Simple Error Handler.vi"("error in (no error)"=w832) -> ()  [unwired: 4 in, 5 out]
    }
  }
  "BW icon out" <- w56
  "Error code out" <- w61
  "Color icon out" <- w37
  "LabVIEW Icon out" <- w30
